vi "Text control 2 v7.1.vi"() -> ()   [LabVIEW 2016]
panel:
  in  "Tab Control":enum32{"Main", "Other parameters"}(tab)
  in  "Plot sample extrema vs time":bool
  out "Line running":i32
  out "Total lines":i32
  out "Path":path=path "C:/users/rlp38/09Apr2009LTtesting/test2.txt"
  out "I vs Vg":cluster{"Y data in":dbl[], "X data in":dbl[]}[](graph)
  out "Is max":dbl format="%.2e"
  out "Id max":dbl format="%.2e"
  out "Ig max":dbl format="%.2e"
  out "Imax vs time":cluster{"Y data in":dbl[], "X data in":dbl[]}[](graph)
  out "Imin vs time":cluster{"Y data in":dbl[], "X data in":dbl[]}[](graph)
  out "I vs Vd":cluster{"Y data in":dbl[], "X data in":dbl[]}[](graph)
  in  "Script":string="#pulsedstressV d 0.03 20 0 0.5 0.0827 5\n#\n#itime m\n#gaterangemode a\n#drainrangemode a\n#pulsed on 0.05 0 0.02\n#transfer d -10 40 1 5 40 35\n#transfer d -10 40 1 5 40 35\n#transfer d -10 40 1 5 40 35\n#output d 0 40 20 0 40 1\n#\n#\n#sample 1 0.008 221 6 0.003\n#samplei 400e-6 200 6 0.002 0.1\n#vsu2pulse -10 4\n#\n#stressV 0.016 0.03 2e-4 0.1e-3 11\n#stressI 220e-7 0.08 15\n#transfer s -1 1 0.5 -0.005 0.005 0.005\n#output s 0 0 0 -0.008 0.008 0.002"
  out "Command running:":string
  out "Serial port data":string
  out "Elapsed Time":dbl caption="Elapsed Time (s)"
  in  "Time Units":u16(ring)=1 items=["Seconds", "Minutes", "Hours"]
  in  "Time Offset":dbl caption="Set Start Time (s)"
  in  "Reset":bool
  in  "Auto Reset":bool
  in  "integration time":u32(slide) max=2 step=1 scale=0.0..2.0
  out "Is on":dbl format="%.2e"
  out "Id on":dbl format="%.2e"
  out "Ig on":dbl format="%.2e"
  out "Ion vs time":cluster{"Y data in":dbl[], "X data in":dbl[]}[](graph)
  out "Ioff vs time":cluster{"Y data in":dbl[], "X data in":dbl[]}[](graph)
  out "Ig min":dbl format="%.2e"
  out "Id min":dbl format="%.2e"
  out "Is min":dbl format="%.2e"
  out "Is off":dbl format="%.2e"
  out "Id off":dbl format="%.2e"
  out "Ig off":dbl format="%.2e"
  in  "Integration time (long)":dbl=0.32 min=0.04 max=2.0 step=0.02 format="%.2f"
  in  "Integration time (short)":dbl=0.0019 min=8e-05 max=0.0019 step=8e-05 format="%^.0e"
  in  "Drain: Compliance":dbl=0.001 format="%.8f"
  in  "Gate: Compliance":dbl=0.001 format="%.8f"
  in  "Interrupt scan":bool
  in  "Interrupt program":bool
  in  "Plot output curve extrema vs time":bool
  in  "Plot transfer curve extrema vs time":bool
  out "I vs time (Bias Stress)":cluster{"Y data in":dbl[], "X data in":dbl[]}[](graph)
  in  "Sample I - Probe 4 (Disabled)":u32(ring)=3 items=["SMU1  ", "SMU2  ", "SMU3  ", "SMU4  ", "SMU5  ", "SMU6  ", "VSU1  ", "VSU2  "]
  in  "Sample I - Source/Common":u32(ring) items=["SMU1  ", "SMU2  ", "SMU3  ", "SMU4  ", "SMU5  ", "SMU6  ", "VSU1  ", "VSU2  "]
  in  "Sample I - Probe 3 (Disabled)":u32(ring)=2 items=["SMU1  ", "SMU2  ", "SMU3  ", "SMU4  ", "SMU5  ", "SMU6  ", "VSU1  ", "VSU2  "]
  in  "Sample I - Drain/Gate":u32(ring)=1 items=["SMU1  ", "SMU2  ", "SMU3  ", "SMU4  ", "SMU5  ", "SMU6  ", "VSU1  ", "VSU2  "]
  in  "Sample - Probe 4":u32(ring)=3 items=["SMU1  ", "SMU2  ", "SMU3  ", "SMU4  ", "SMU5  ", "SMU6  ", "VSU1  ", "VSU2  "]
  in  "Sample - Source/Common":u32(ring) items=["SMU1  ", "SMU2  ", "SMU3  ", "SMU4  ", "SMU5  ", "SMU6  ", "VSU1  ", "VSU2  "]
  in  "Sample - Gate":u32(ring)=2 items=["SMU1  ", "SMU2  ", "SMU3  ", "SMU4  ", "SMU5  ", "SMU6  ", "VSU1  ", "VSU2  "]
  in  "Sample - Drain":u32(ring)=1 items=["SMU1  ", "SMU2  ", "SMU3  ", "SMU4  ", "SMU5  ", "SMU6  ", "VSU1  ", "VSU2  "]
  in  "Gate Range\nmode":u16(ring) items=["Auto", "Limited", "Fixed"]
  in  "Gate Range":u8(slide)=3 max=11 scale=0.0..11.0
  in  "Source/Drain\nRange mode":u16(ring) items=["Auto", "Limited", "Fixed"]
  in  "Source/Drain Range":u8(slide)=3 max=11 scale=0.0..11.0
  in  "Panel Controls":T1={"Emergency Stop"=refnum, "TransGraph Max"=1e-05, "Text/Graph (text=false)"=TRUE} {"TransGraph Max" format="%.2e"}
  in  "Panel Controls 2":T2={"Emergency Stop"=refnum, "TransGraph Max"=1e-05, "Text/Graph (text=false)"=TRUE, "TransGraph Min"=1e-11} {"TransGraph Min" format="%.2e"; "TransGraph Max" format="%.2e"}
  out "error out":errorcluster
  in  "Delay before read (ms)":u32=1000
  in  "byte count":u32=64
  in  "Serial End Mode for Reads":u16(ring)=2 items=["None", "LastBit", "TermChar"]
  in  "Timeout (ms)":u32=10000
  in  "Enable Termination\nChar (T)":bool=TRUE
  in  "Termination char\n(0xA = '\\n' = LF)\n(0xD = '\\r' = CR)":u8=13 format="%.0x"
  in  "flow control":u16(ring) items=["None"=0, "XON/XOFF"=1, "RTS/CTS"=2, "DTR/DSR"=4]
  in  "stop bits":u16(ring)=10 items=["1.0"=10, "1.5"=15, "2.0"=20]
  in  "parity":u16(ring) items=["None", "Odd", "Even", "Mark", "Space"]
  in  "data bits":u16=8 min=5 max=8 step=1
  in  "VISA resource name":refnum<visa-resource-name>="COM6"
  in  "baud rate":u32=9600
  out "Timings Indicator":T3
  in  "Timings (overwritten by the Front Panel)":T4={"integration time"=0, "Short/Long integration time"=0.00064, "hold time (sec)"=0.0, "delay time (sec)"=0.0, "Step Time (0 disables)"=0.0, "sweep method"=0, "Pulse period"=0.005, "Base voltage"=0.0, "Pulse width"=0.0005} {"Pulse width" min=0.0005 max=0.1 step=0.0001 format="%.4f"; "Base voltage" format="%^.4e"; "Pulse period" min=0.005 max=1.0 step=0.0001 format="%.4f"; "sweep method" items=["Continuous", "Pulsed"]; "Step Time (0 disables)" format="%.2f"; "delay time (sec)" format="%.4f"; "hold time (sec)" format="%.4f"; "Short/Long integration time" format="%^.0e"; "integration time" scale=0.0..2.0}
  in  "Probe 4":cluster{"on/off":bool, "Voltage":dbl} {"Voltage" min=-100.0 max=100.0 format="%.2f"}
  in  "Full Reset":bool
  in  "Standby":T5
  out "Probe 4 Indicator":cluster{"on/off":bool, "Voltage":dbl} {"Voltage" min=-100.0 max=100.0 format="%.2f"}
  in  "Transfer/Output - Drain":u32(ring)=1 items=["SMU1  ", "SMU2  ", "SMU3  ", "SMU4  ", "SMU5  ", "SMU6  ", "VSU1  ", "VSU2  "]
  in  "Transfer/Output - Gate":u32(ring)=2 items=["SMU1  ", "SMU2  ", "SMU3  ", "SMU4  ", "SMU5  ", "SMU6  ", "VSU1  ", "VSU2  "]
  in  "Transfer/Output - Source/Common":u32(ring) items=["SMU1  ", "SMU2  ", "SMU3  ", "SMU4  ", "SMU5  ", "SMU6  ", "VSU1  ", "VSU2  "]
  in  "Transfer/Output - Probe 4":u32(ring)=3 items=["SMU1  ", "SMU2  ", "SMU3  ", "SMU4  ", "SMU5  ", "SMU6  ", "VSU1  ", "VSU2  "]
  in  "Pulsed Stress V - Probe 4":u32(ring)=3 items=["SMU1  ", "SMU2  ", "SMU3  ", "SMU4  ", "SMU5  ", "SMU6  ", "VSU1  ", "VSU2  "]
  in  "Pulsed Stress V - Vextra":u32(ring)=7 items=["SMU1  ", "SMU2  ", "SMU3  ", "SMU4  ", "SMU5  ", "SMU6  ", "VSU1  ", "VSU2  "]
  in  "Pulsed Stress V - Drain":u32(ring)=1 items=["SMU1  ", "SMU2  ", "SMU3  ", "SMU4  ", "SMU5  ", "SMU6  ", "VSU1  ", "VSU2  "]
  in  "Pulsed Stress V - Source/Common":u32(ring) items=["SMU1  ", "SMU2  ", "SMU3  ", "SMU4  ", "SMU5  ", "SMU6  ", "VSU1  ", "VSU2  "]
  in  "Pulsed Stress V - Gate":u32(ring)=2 items=["SMU1  ", "SMU2  ", "SMU3  ", "SMU4  ", "SMU5  ", "SMU6  ", "VSU1  ", "VSU2  "]
  in  "FPP - Drain":u32(ring)=1 items=["SMU1  ", "SMU2  ", "SMU3  ", "SMU4  ", "SMU5  ", "SMU6  ", "VSU1  ", "VSU2  "]
  in  "FPP - Gate":u32(ring)=2 items=["SMU1  ", "SMU2  ", "SMU3  ", "SMU4  ", "SMU5  ", "SMU6  ", "VSU1  ", "VSU2  "]
  in  "FPP - Probe 1":u32(ring) items=["SMU1  ", "SMU2  ", "SMU3  ", "SMU4  ", "SMU5  ", "SMU6  ", "VSU1  ", "VSU2  "]
  in  "FPP - Probe 2":u32(ring)=3 items=["SMU1  ", "SMU2  ", "SMU3  ", "SMU4  ", "SMU5  ", "SMU6  ", "VSU1  ", "VSU2  "]
  in  "FPP - Source":u32(ring)=6 items=["SMU1  ", "SMU2  ", "SMU3  ", "SMU4  ", "SMU5  ", "SMU6  ", "VSU1  ", "VSU2  "]
  in  "Stress V - Drain":u32(ring)=1 items=["SMU1  ", "SMU2  ", "SMU3  ", "SMU4  ", "SMU5  ", "SMU6  ", "VSU1  ", "VSU2  "]
  in  "Stress V - Gate":u32(ring)=2 items=["SMU1  ", "SMU2  ", "SMU3  ", "SMU4  ", "SMU5  ", "SMU6  ", "VSU1  ", "VSU2  "]
  in  "Stress V - Source/Common":u32(ring) items=["SMU1  ", "SMU2  ", "SMU3  ", "SMU4  ", "SMU5  ", "SMU6  ", "VSU1  ", "VSU2  "]
  in  "Stress I - Drain/Gate":u32(ring)=1 items=["SMU1  ", "SMU2  ", "SMU3  ", "SMU4  ", "SMU5  ", "SMU6  ", "VSU1  ", "VSU2  "]
  in  "Stress I - Source/Common":u32(ring) items=["SMU1  ", "SMU2  ", "SMU3  ", "SMU4  ", "SMU5  ", "SMU6  ", "VSU1  ", "VSU2  "]
  in  "VSU2 Stress - Source/Common":u32(ring) items=["SMU1  ", "SMU2  ", "SMU3  ", "SMU4  ", "SMU5  ", "SMU6  ", "VSU1  "]
  in  "VISA resource name in":refnum<visa-resource-name>="GPIB0::14::INSTR"
  in  "Gate":T6={"Gate Start"=0.0, "Gate Stop"=2.0, "Gate Step (linear only)"=1.0, "Gate Compliance"=0.0001, "Gate PComp"=0.0, "Range mode"=0, "Range"=6} {"Range" max=11 scale=0.0..11.0; "Range mode" items=["Auto", "Limited", "Fixed"]; "Gate PComp" format="%^.2e"; "Gate Compliance" format="%^.2e"; "Gate Step (linear only)" format="%^.4e"; "Gate Stop" format="%^.4e"; "Gate Start" format="%^.4e"}
  in  "Drain 2":T7={"Drain Start"=0.0, "Drain Stop"=2.0, "Drain Compliance"=0.0001, "Drain Step"=1.0, "Drain PComp"=0.0, "Range mode"=0, "Range"=6} {"Range" max=11 scale=0.0..11.0; "Range mode" items=["Auto", "Limited", "Fixed"]; "Drain PComp" format="%^.2e"; "Drain Step" format="%^.4e"; "Drain Compliance" format="%^.2e"; "Drain Stop" format="%^.4e"; "Drain Start" format="%^.4e"}
  # "Time"
  # "Syntax:\nitime [s|m|l] time(sec): [s|m|l] determines the integration time setting (small|medium|long) and time sets the value.\nNOTE: The value of the integration time has to be within the range allowed by its category (s|m|l), otherwise, the closest value will be used. (e.g. if the category is set to short but the time value is very long, the actual value used will be the maximum short integration time.\nIntegration times:\n    Short: Default: 640 us. Range: 8E-5 - 1.92E-3 seconds.\n    Medium: Fixed at 1 NPL cycle (0.02 seconds).\n    Long: Default: 16 NPL cycles (0.32 seconds). Range: 2-100 NPL cycles (0.04 seconds - 2 seconds).\ngaterangemode [a|l|f]\ndrainrangemode [a|l|f]\npulsed [on|off] PulsePeriod(sec) PulseBaseVoltage PulseONWidth(sec)\nstandby [on l off]\nwait NumMilliseconds\nwait-min NumMinutes\n# texthere = comment\nProbe4 [ON|OFF] Voltage\ntransfer [s|d] VgStart VgStop VgStep VdStart VdStop VdStep\noutput [s|d] VgStart VgStop VgStep VdStart VdStop VdStep\nsample Vg Vd NumSamples Time(s) SampleInterval(s)\nsamplei Idg NumSamples Time(s) SampleInterval(s) VDGcompliance\n100 samples is approximately 13 seconds with medium integration\n# if in doubt use SampleInterval(s) = 0.004\n    NOTE: When doing bias stress measurements, it is best to set the Time Units to \"Seconds\", as the \"sample\" command has been configured to give the output to seconds.\nstressV VG VD IGcompliance IDcompliance Duration(sec)\nstressI IDG VDGcompliance Duration(sec)\nvsu2pulse Bias Duration(s)\npulsedstressV [s|d] VEstop VgON VgOFF Period(s) PulseONwidth(s) Vd\nsample-fpp Vg Vd NumSamples Time\nresample-fpp Vg Vd\ntransfer-fpp [s|d] VgStart VgStop VgStep VdStart VdStop VdStep\noutput-fpp [s|d] VgStart VgStop VgStep VdStart VdStop VdStep\nserial SerialPortCommand"
  # "1\n2\n3\n4\n5\n6\n7\n8\n9\n10\n11\n12\n13\n14\n15\n16\n17\n18\n19\n20"
  # "SMUs"
  # "Serial port settings"
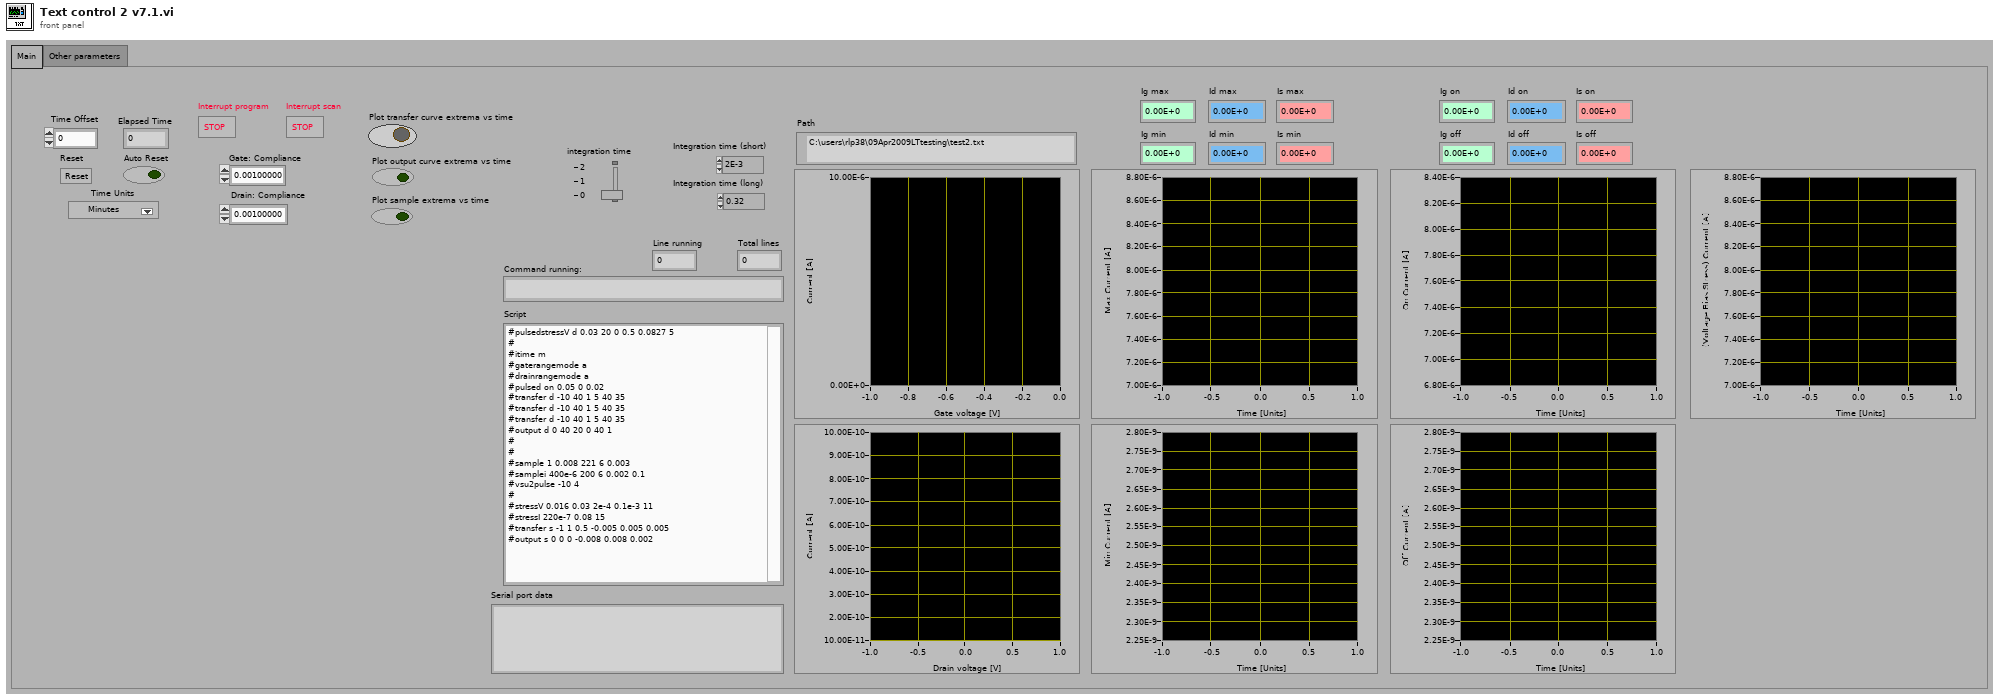
[diagram p1: front panel]
types:
  T1 = cluster{"Emergency Stop":refnum<vi>, "TransGraph Max":dbl, "Text/Graph (text=false)":bool}
  T2 = cluster{"Emergency Stop":refnum<vi>, "TransGraph Max":dbl, "Text/Graph (text=false)":bool, "TransGraph Min":dbl}
  T3 = cluster{"integration time (0:s, 1:m, 2:l)":u32, "Short/Long integration time":dbl, "hold time (sec)":dbl, "delay time (sec)":dbl, "Step Time (0 disables)":dbl, "sweep method":u16, "Pulse period":dbl, "Base voltage":dbl, "Pulse width":dbl}
  T4 = cluster{"integration time":u32, "Short/Long integration time":dbl, "hold time (sec)":dbl, "delay time (sec)":dbl, "Step Time (0 disables)":dbl, "sweep method":u16, "Pulse period":dbl, "Base voltage":dbl, "Pulse width":dbl}
  T5 = cluster{"Gate Standby":bool, "Drain Standby":bool}
  T6 = cluster{"Gate Start":dbl, "Gate Stop":dbl, "Gate Step (linear only)":dbl, "Gate Compliance":dbl, "Gate PComp":dbl, "Range mode":u16, "Range":u8}
  T7 = cluster{"Drain Start":dbl, "Drain Stop":dbl, "Drain Compliance":dbl, "Drain Step":dbl, "Drain PComp":dbl, "Range mode":u16, "Range":u8}
  T8 = enum16{"open", "replace", "create", "open or create", "replace or create", "replace or create with confirmation"}
  T9 = cluster{"V2 Start":dbl, "V2 Step":dbl, "Number of points":i32}
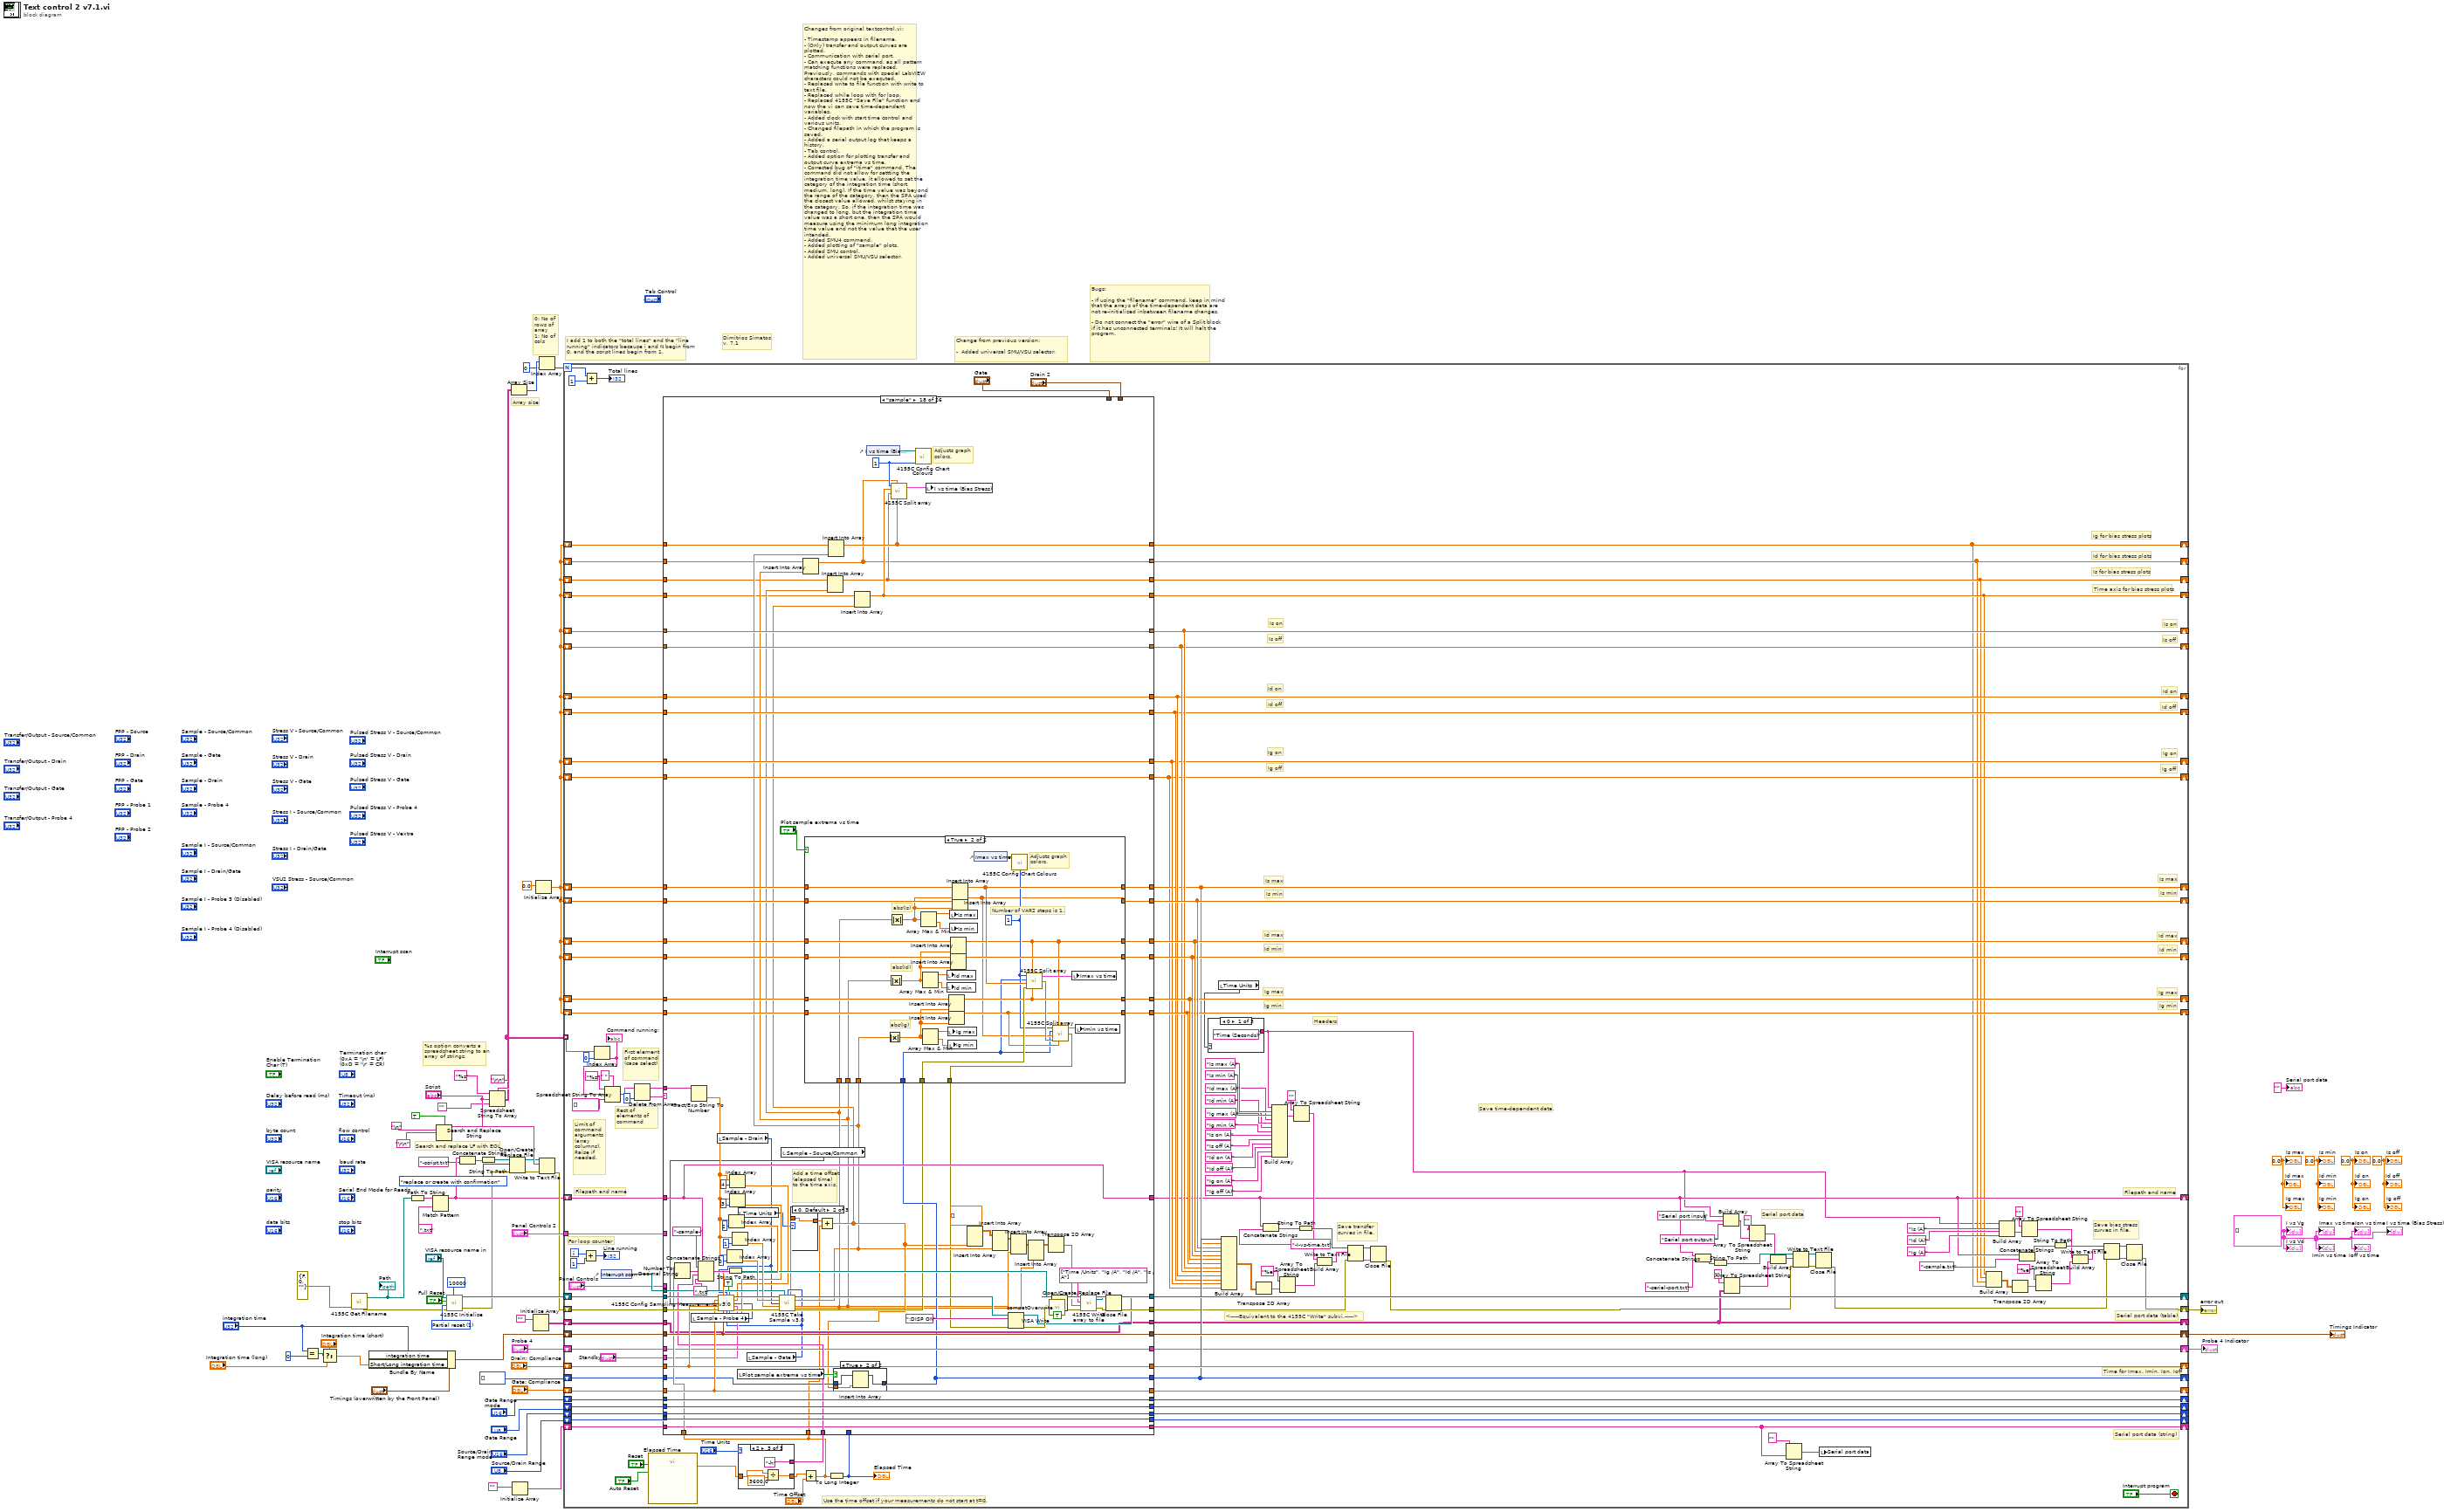
[diagram p0: block diagram]
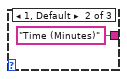
[diagram p2: hidden frame]
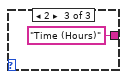
[diagram p3: hidden frame]
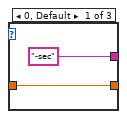
[diagram p4: hidden frame]
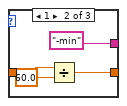
[diagram p5: hidden frame]
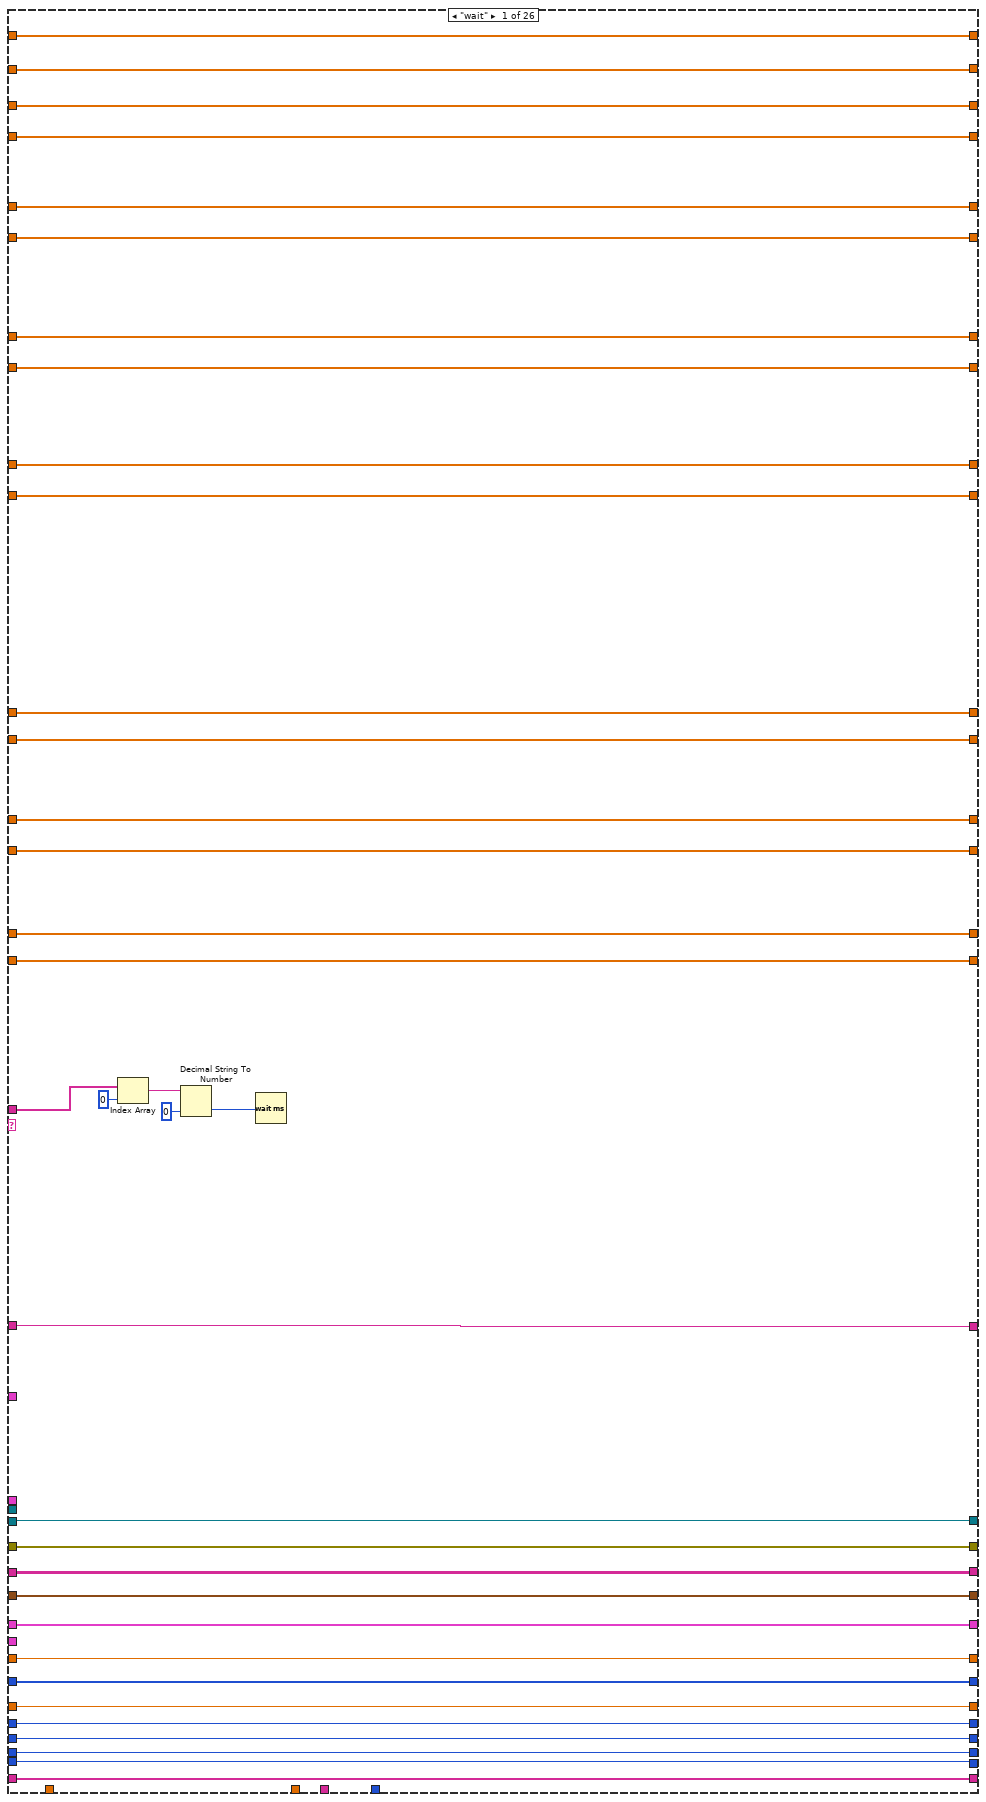
[diagram p6: hidden frame]
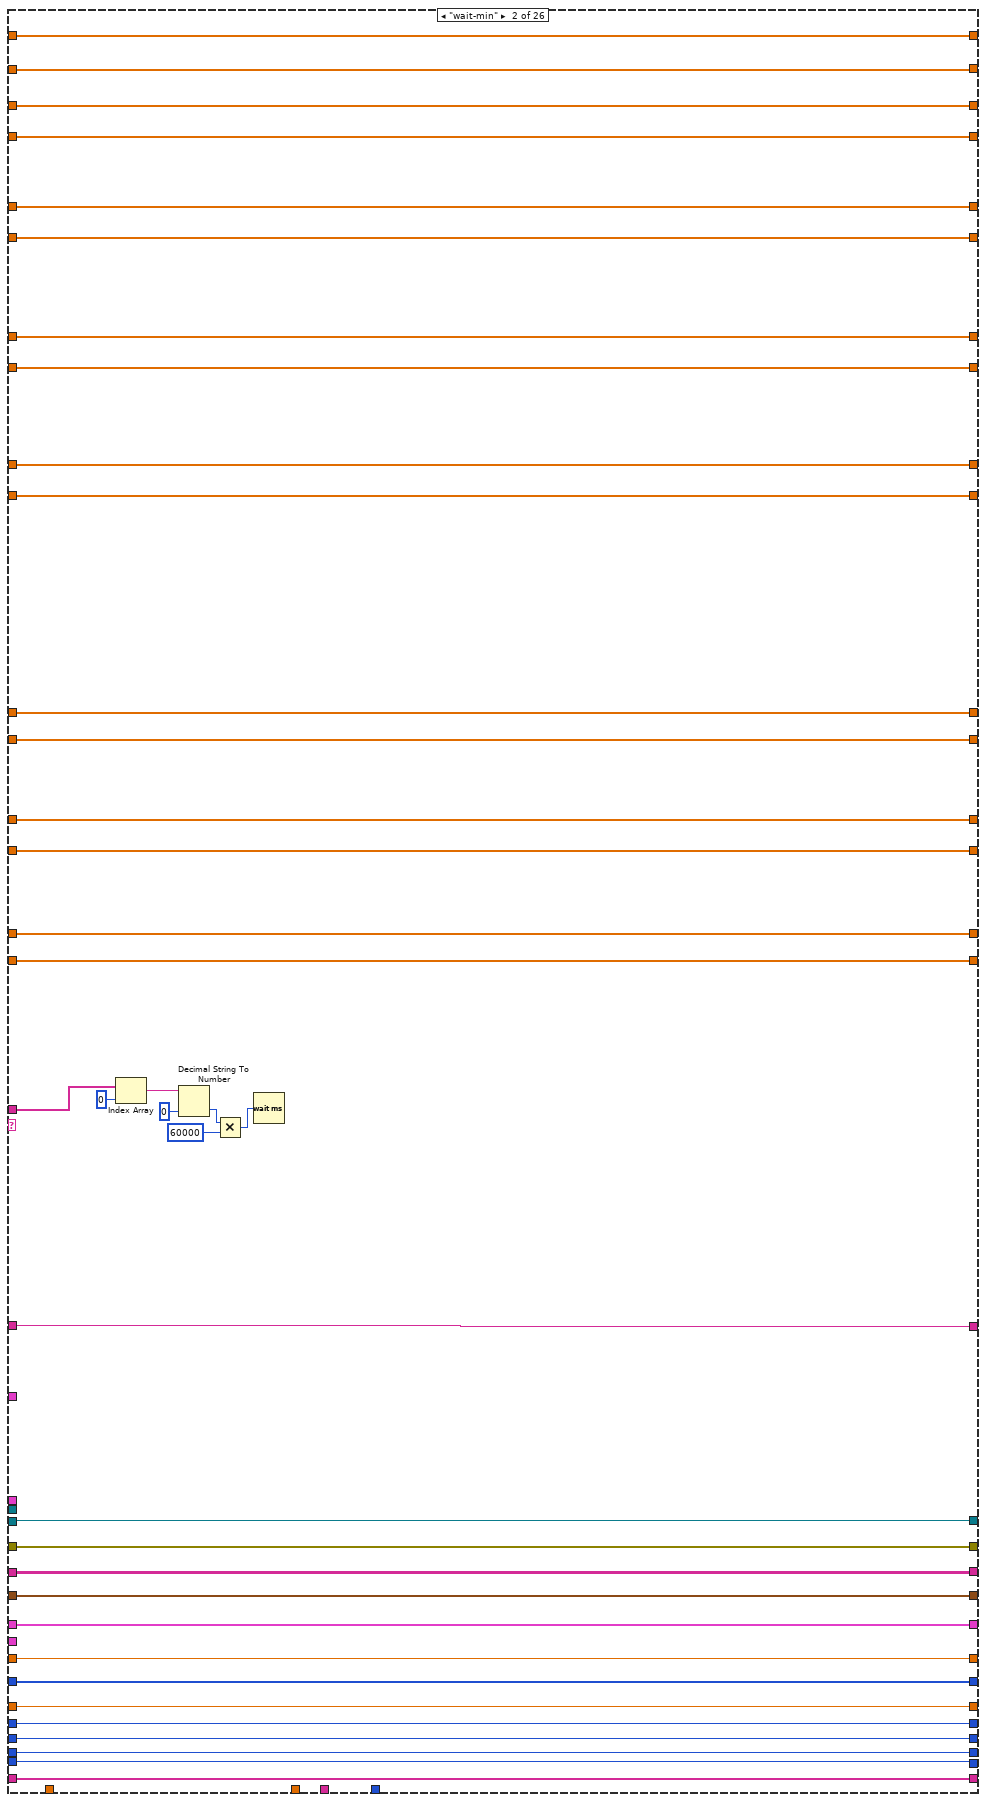
[diagram p7: hidden frame]
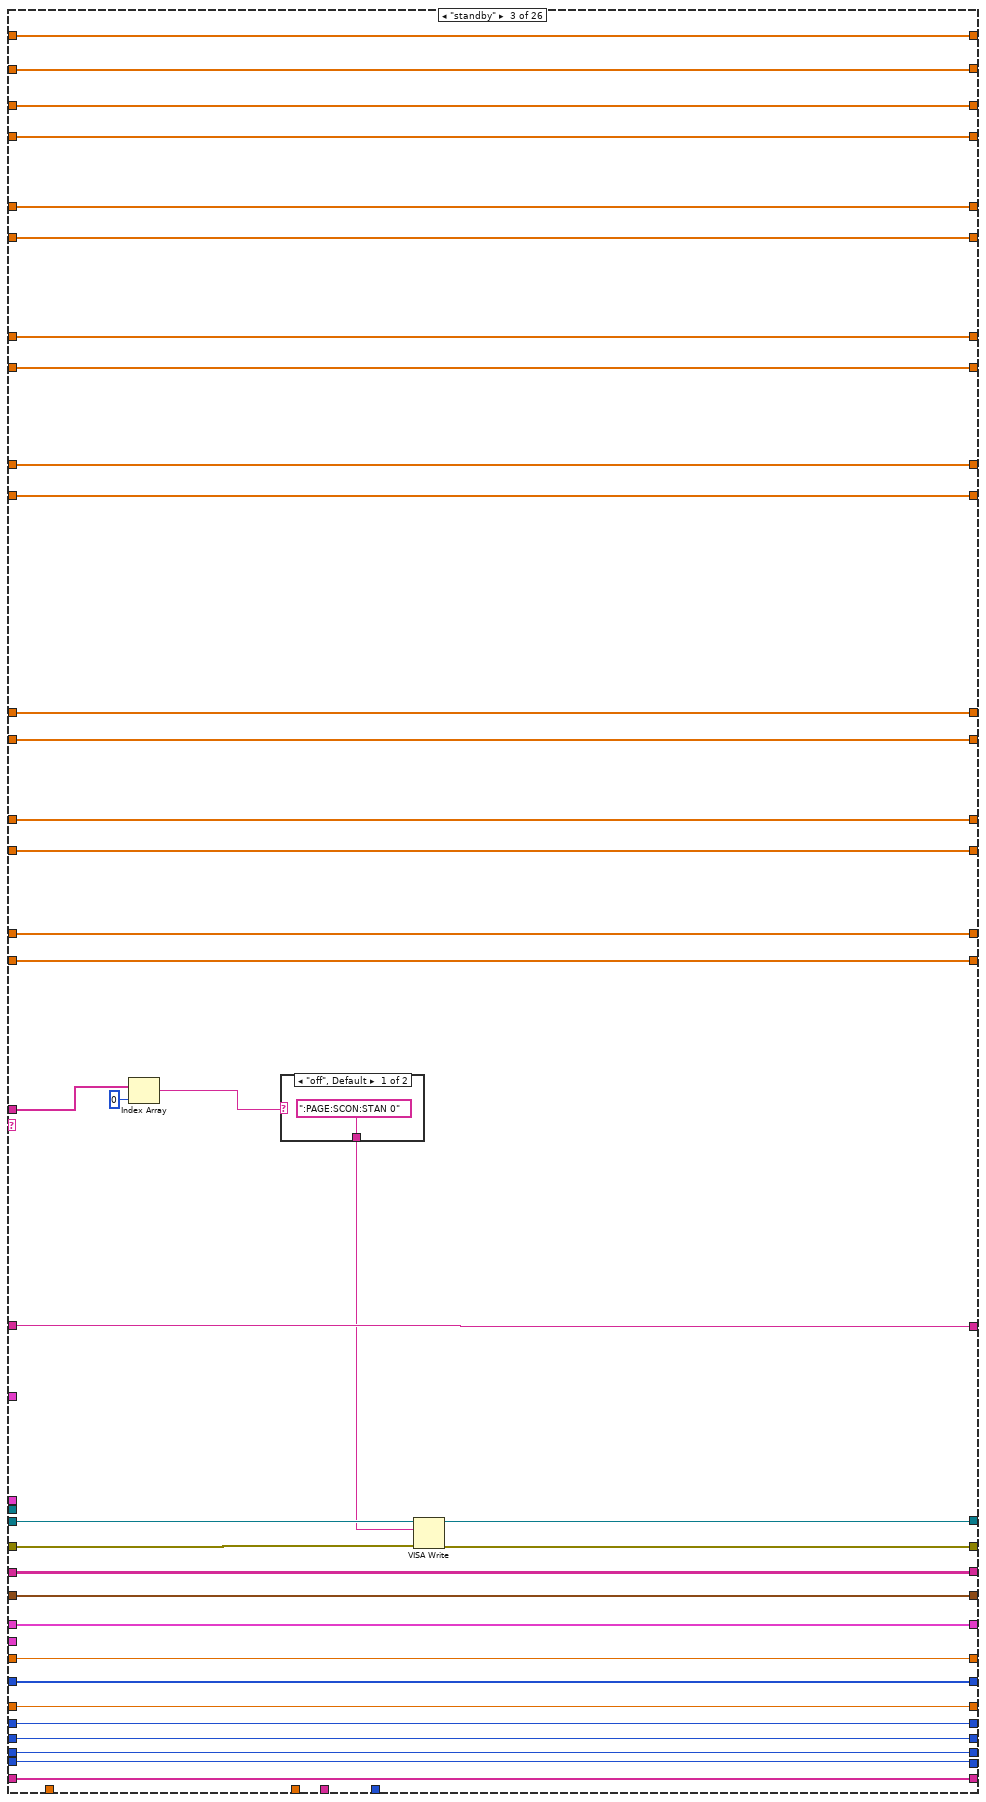
[diagram p8: hidden frame]
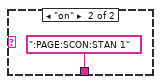
[diagram p9: hidden frame]
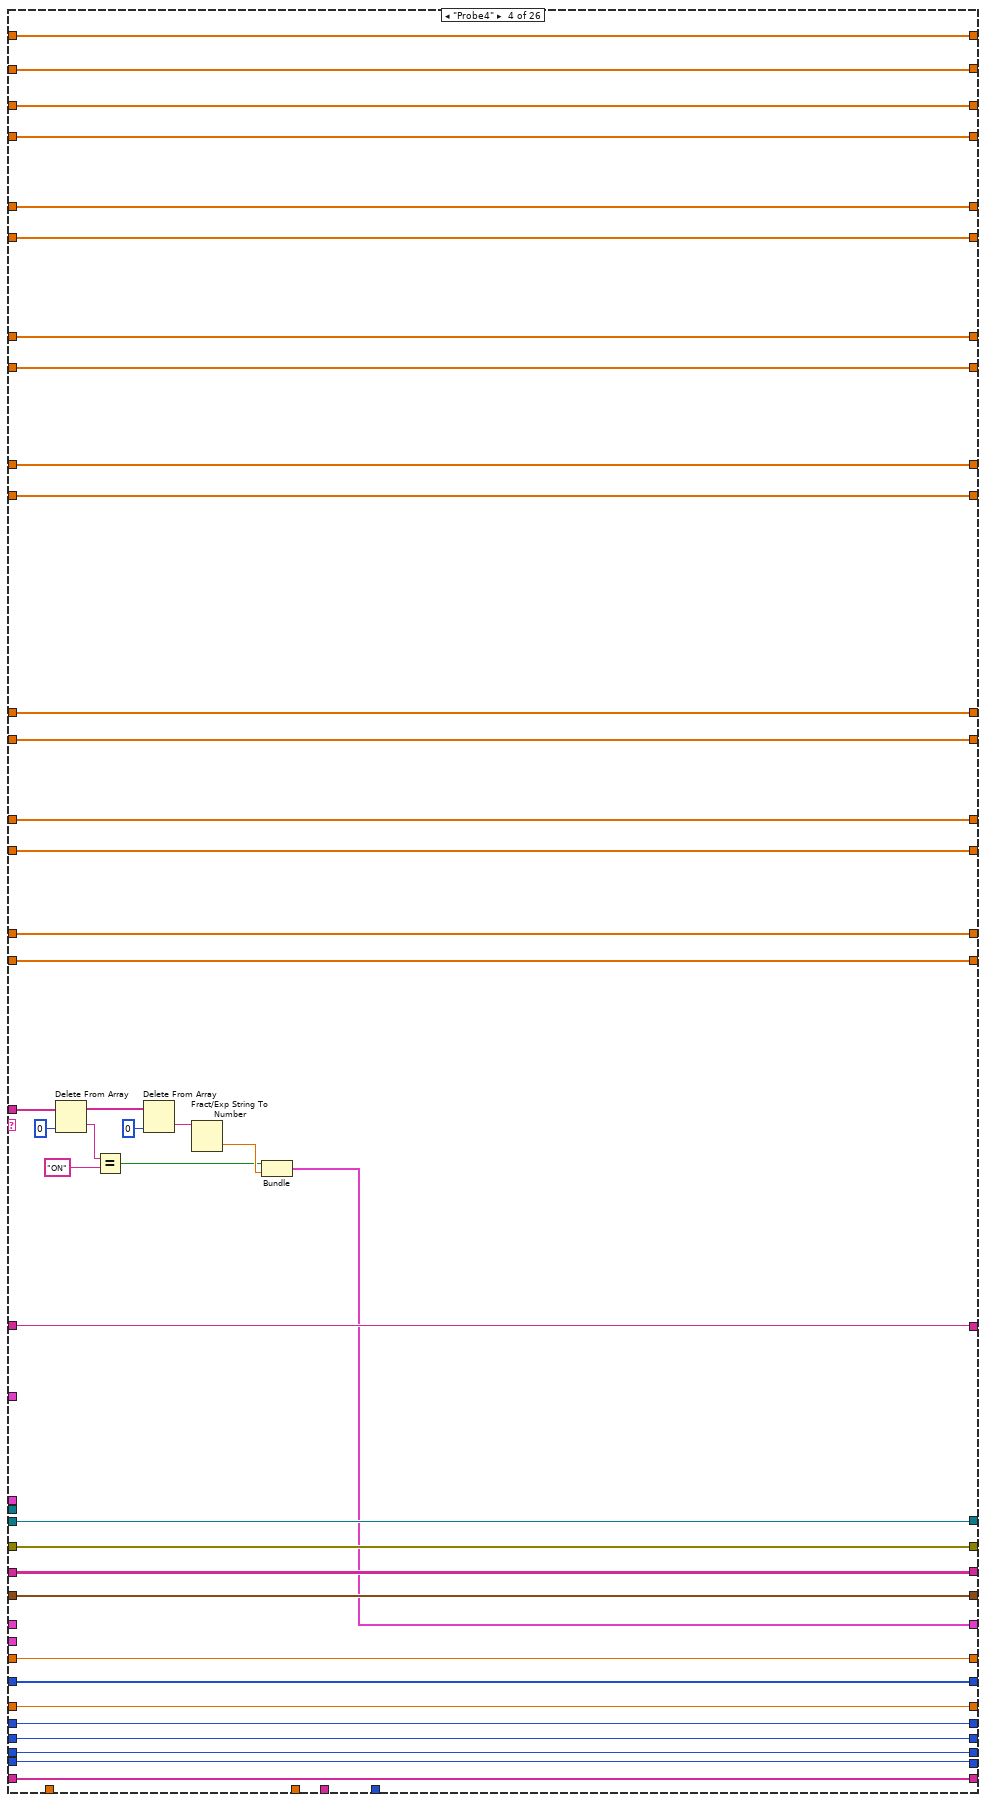
[diagram p10: hidden frame]
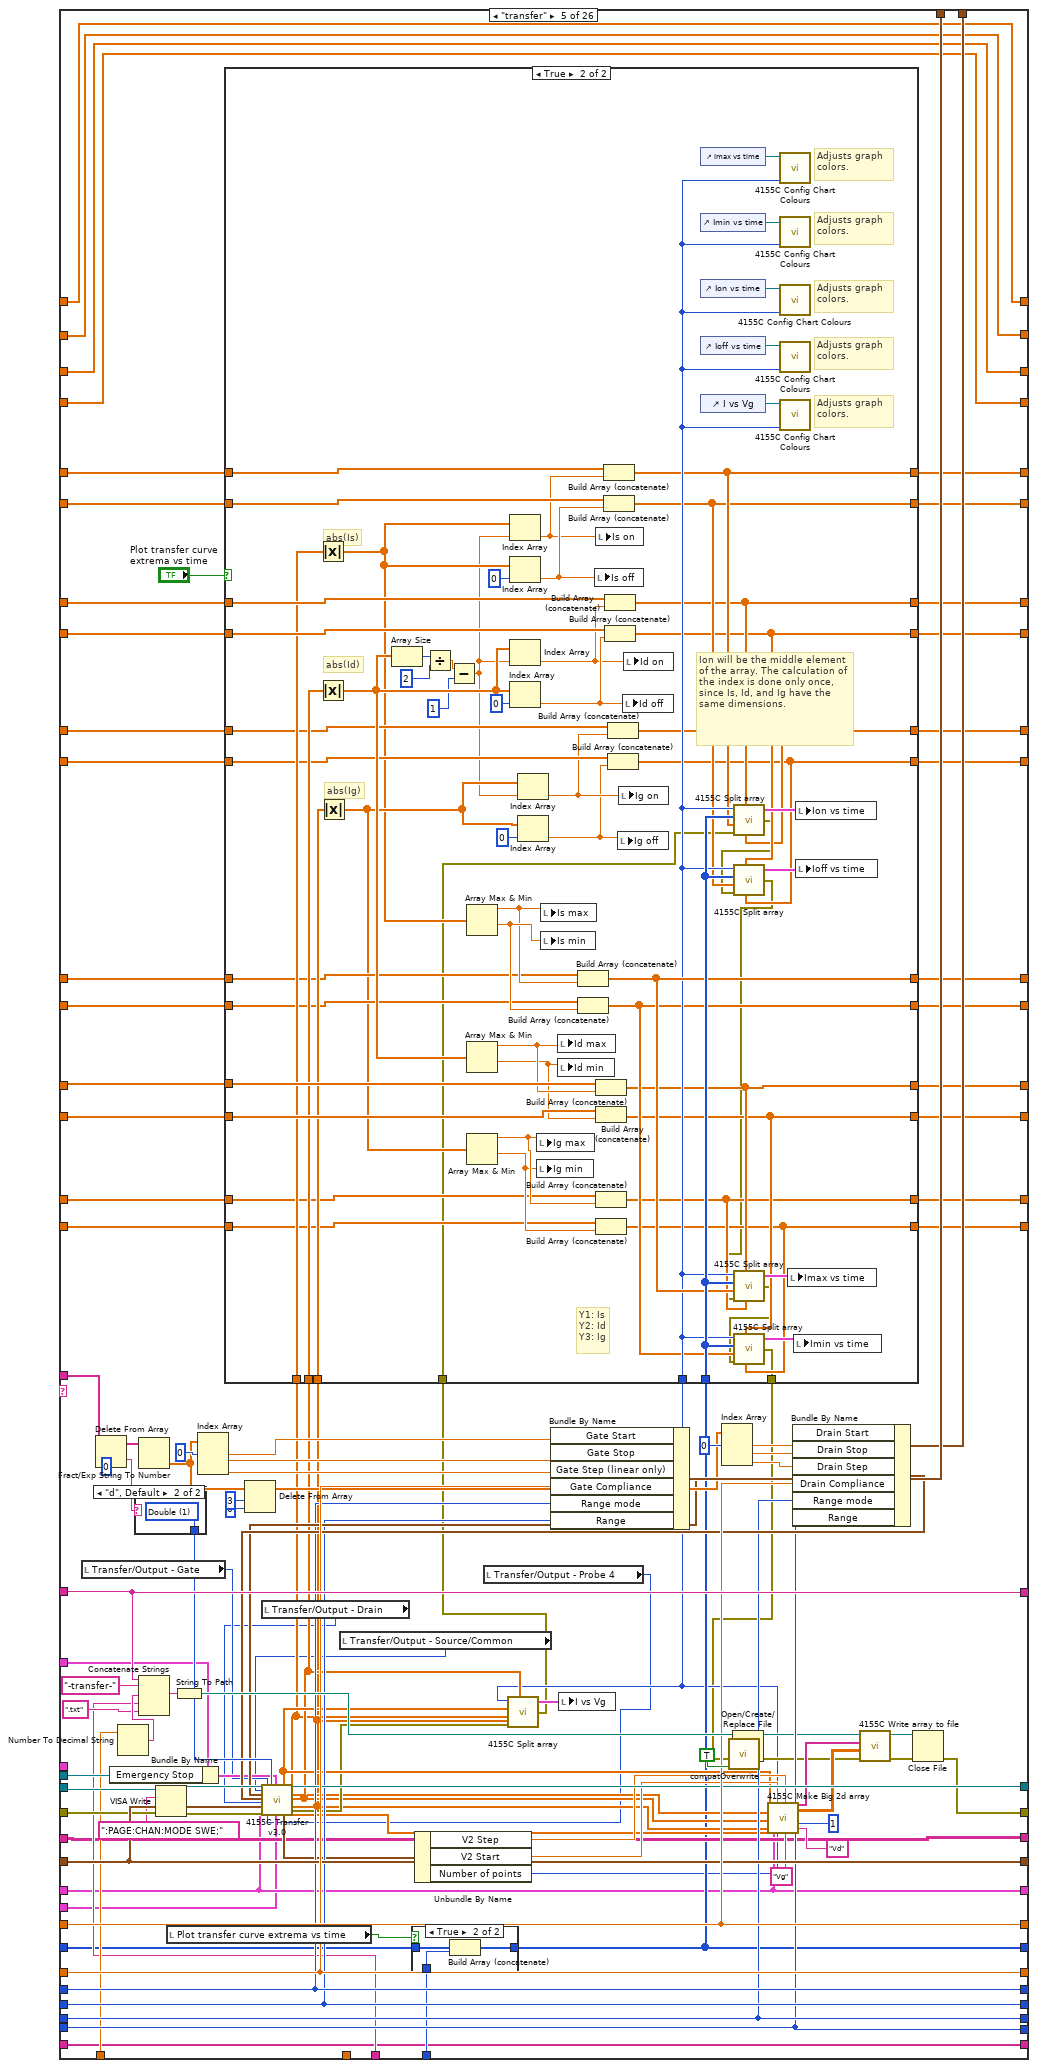
[diagram p11: hidden frame]
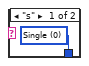
[diagram p14: hidden frame]
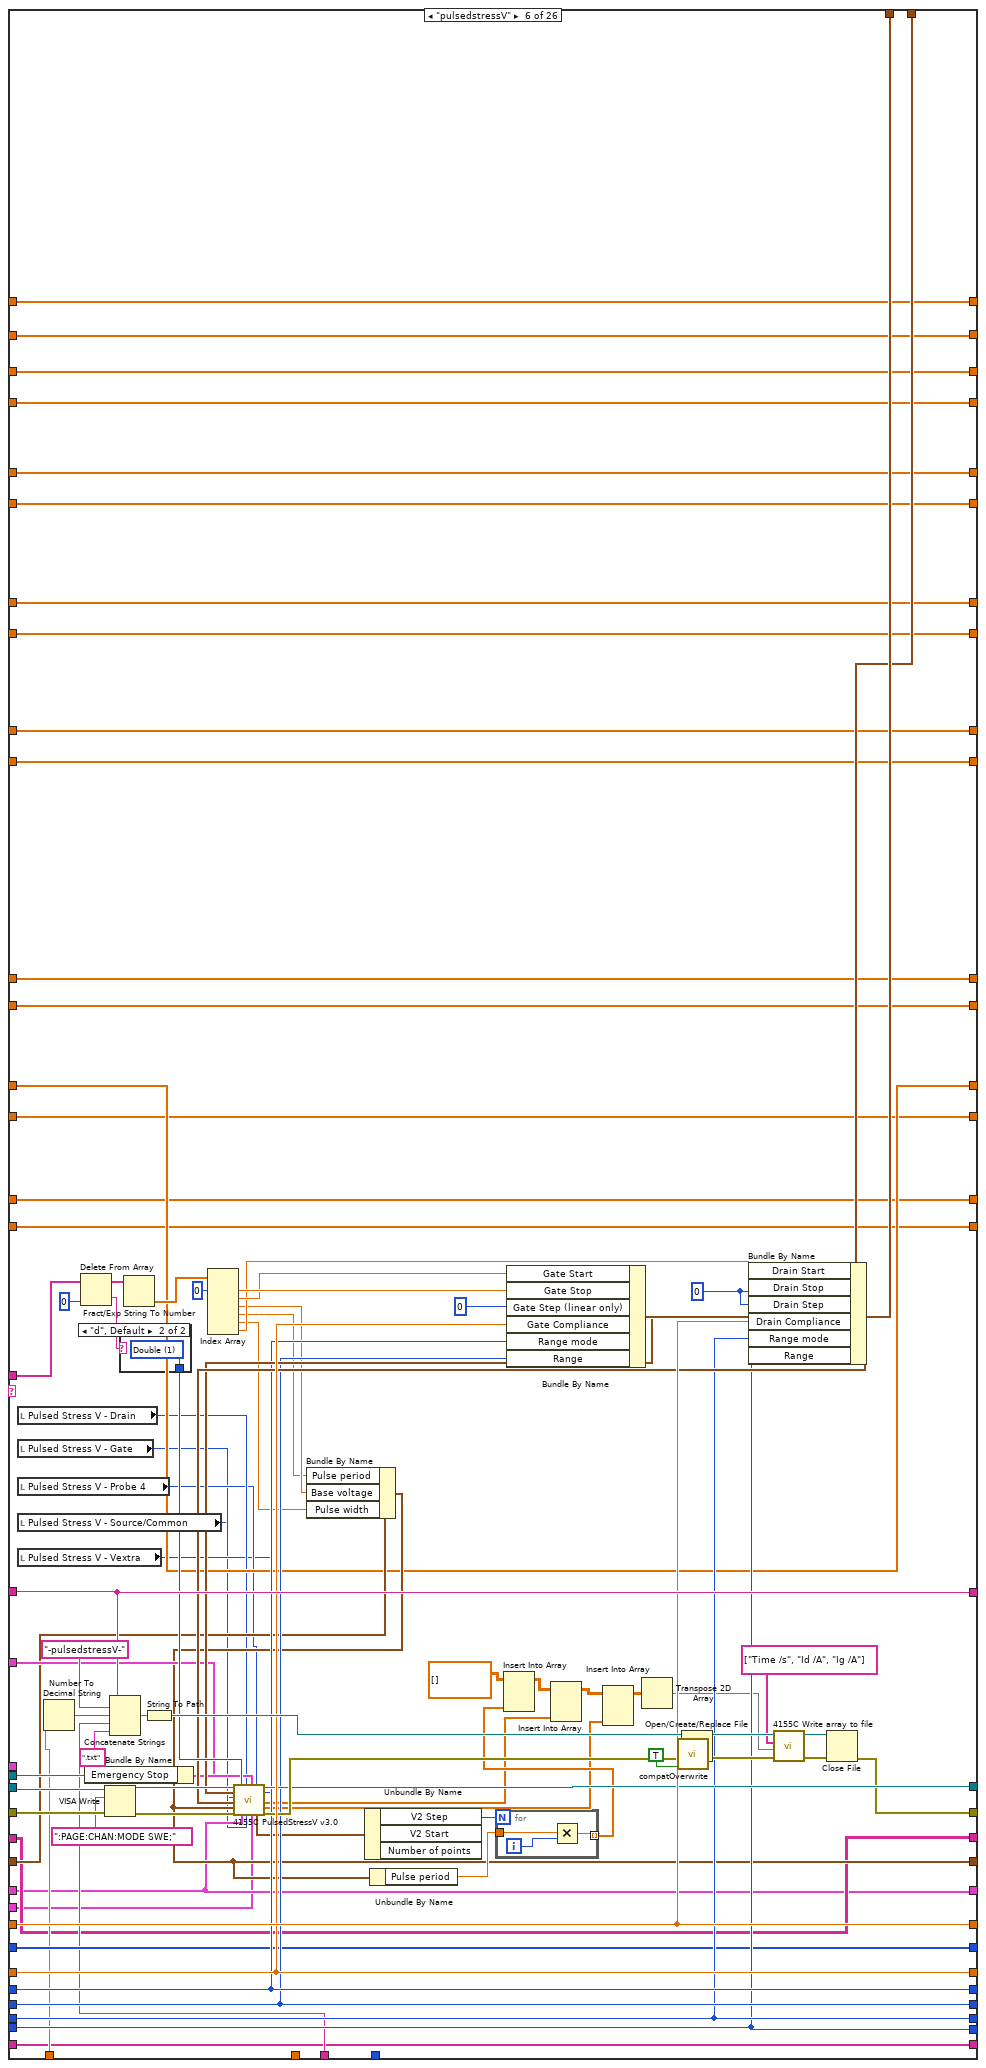
[diagram p15: hidden frame]
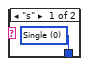
[diagram p16: hidden frame]
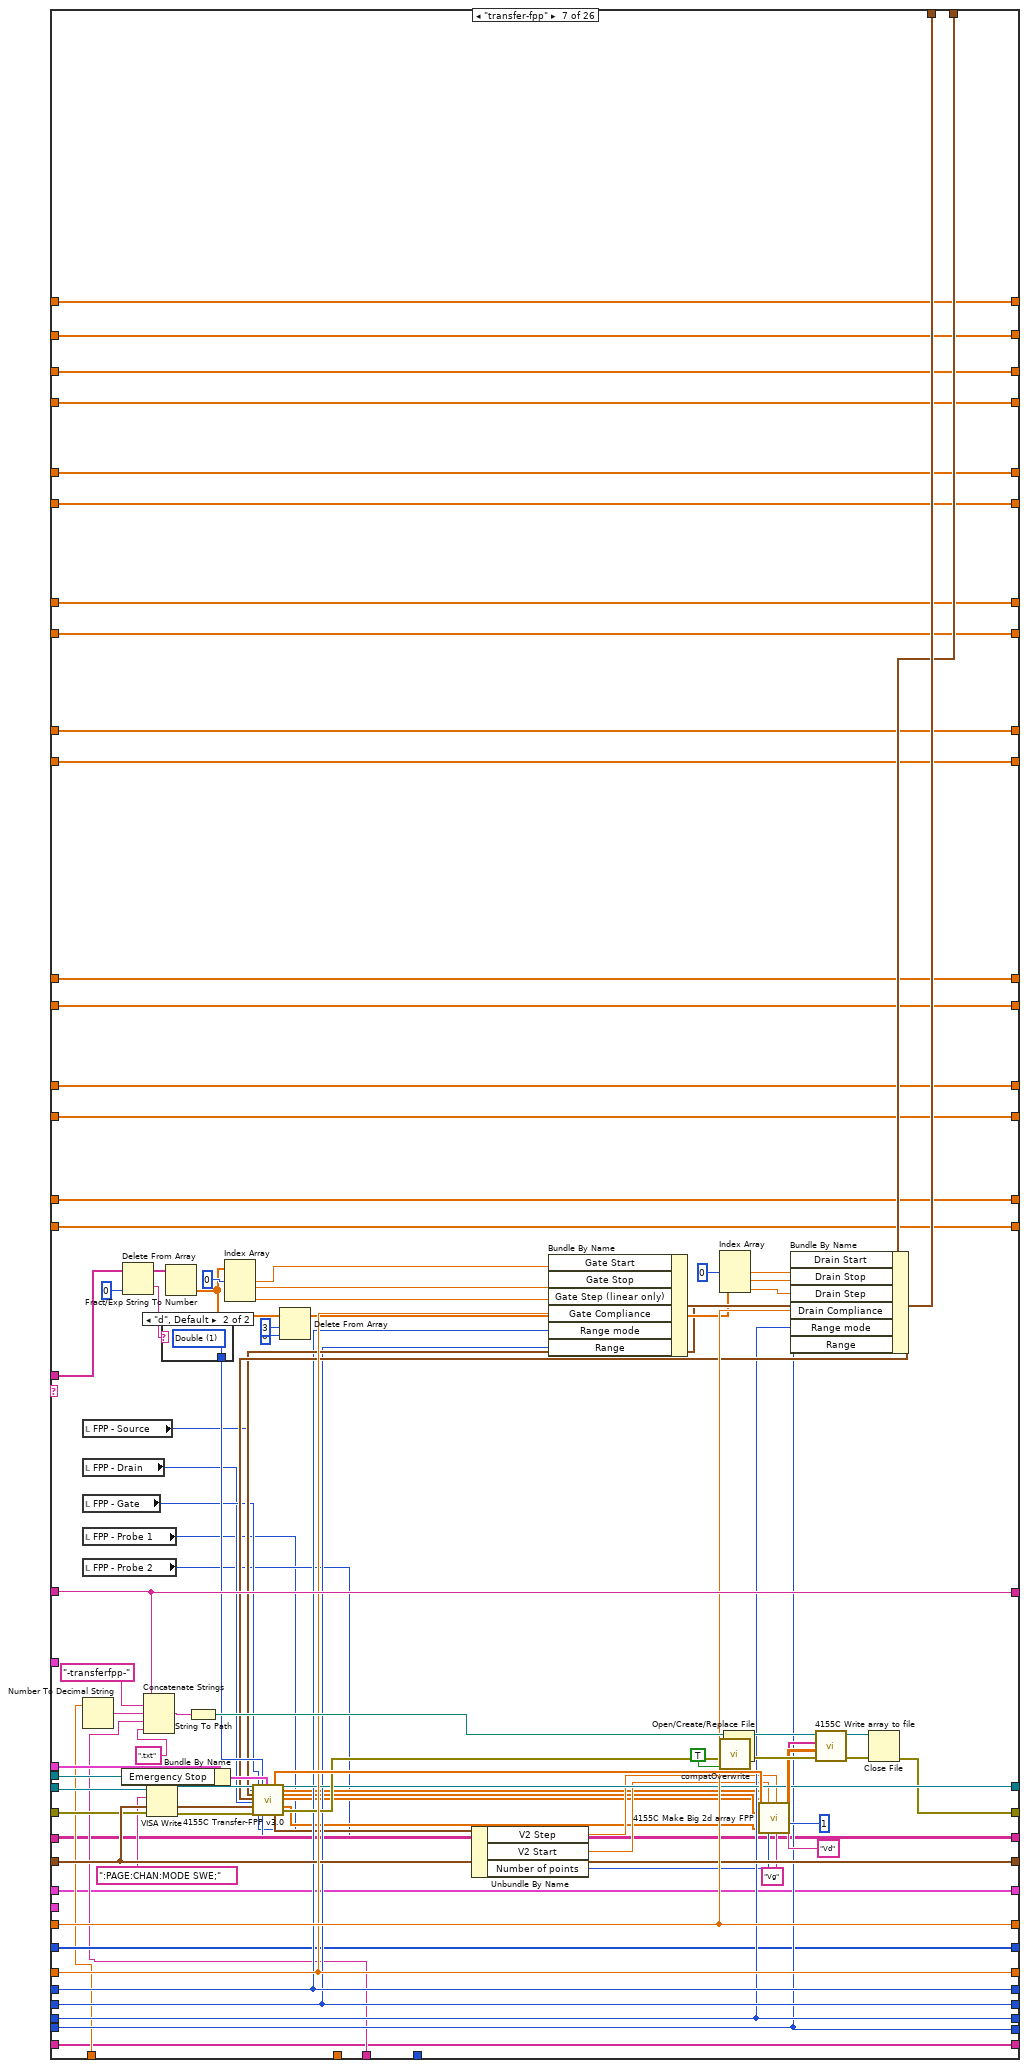
[diagram p17: hidden frame]
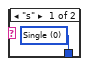
[diagram p18: hidden frame]
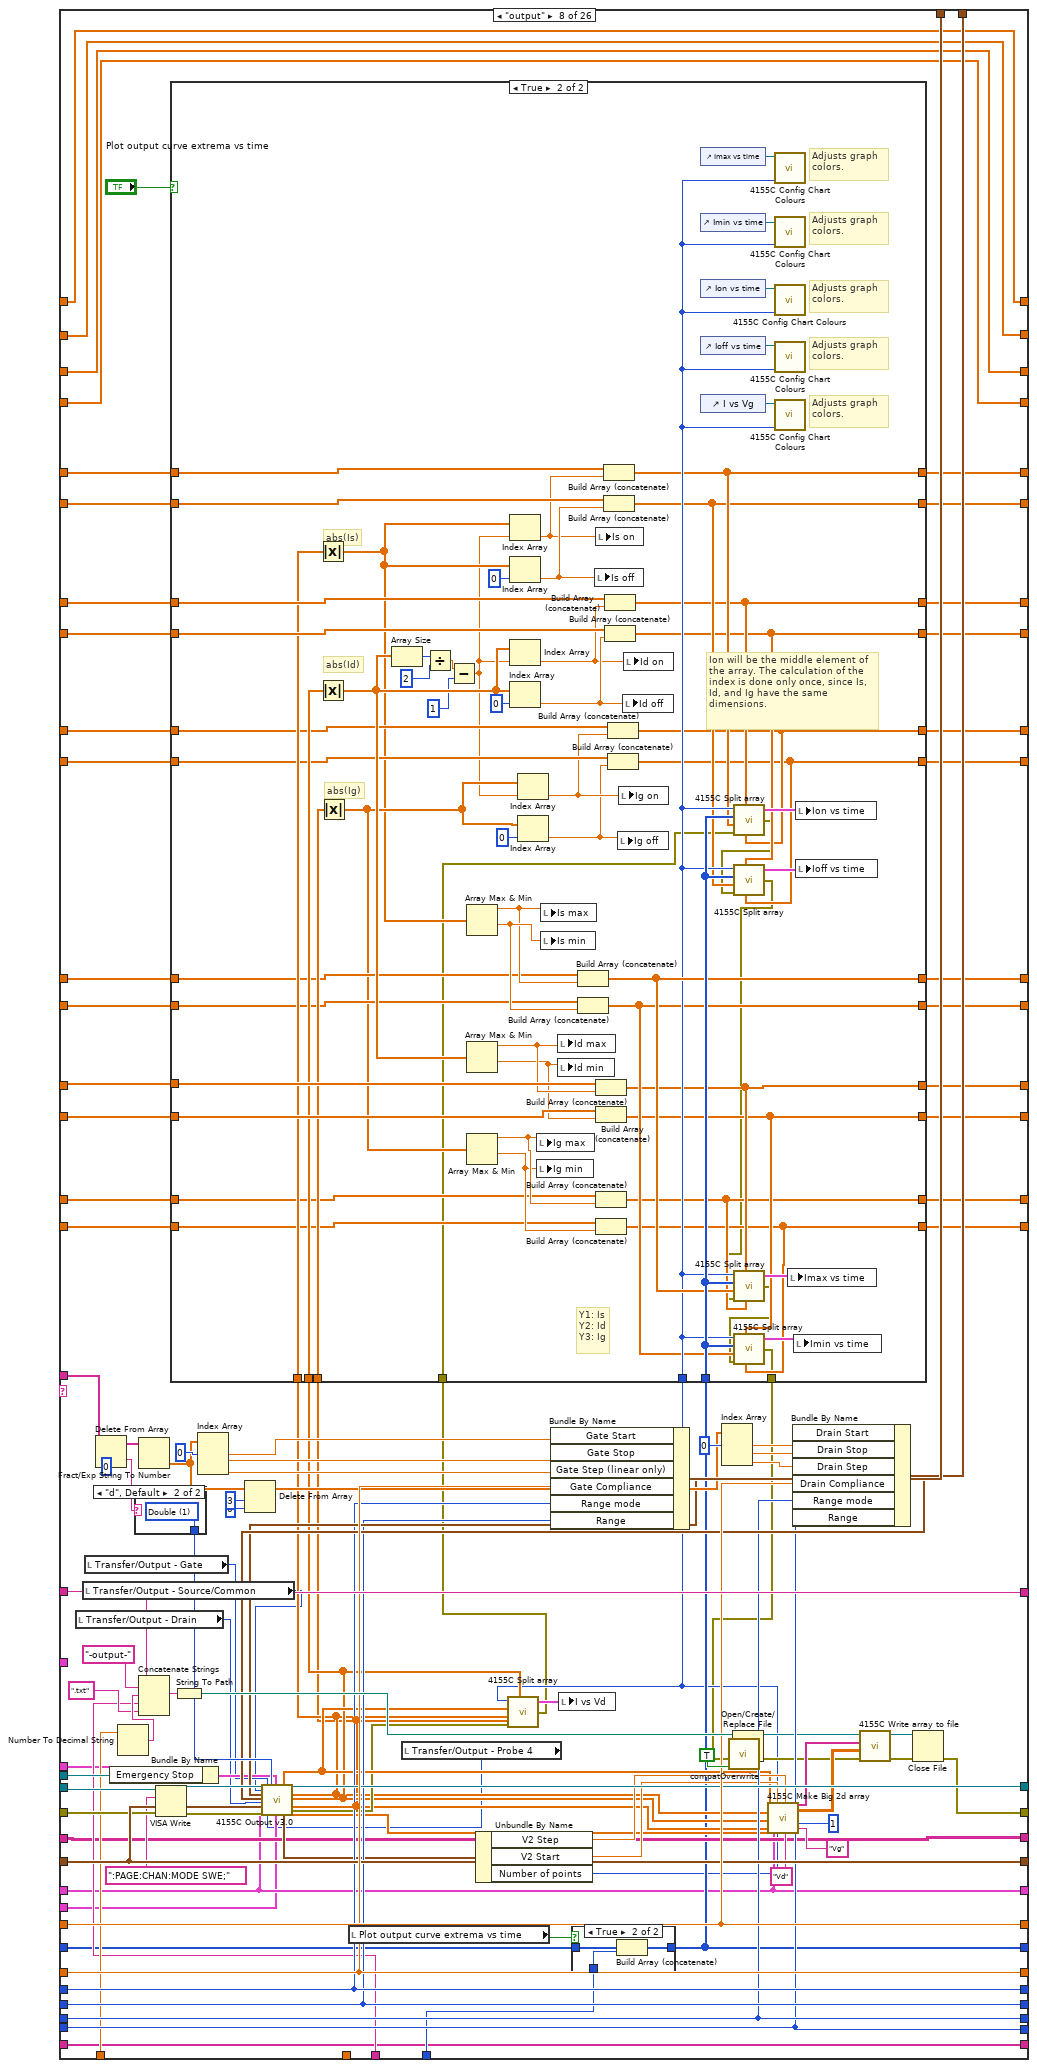
[diagram p19: hidden frame]
diagram:
  w2 = cluster{"Y data in":dbl[], "X data in":dbl[]}[] [] ("I vs Vg")
  w10 = 0.0 ("Is off")
  w11 = 0.0 ("Is on")
  w12 = 0.0 ("Is min")
  w13 = 0.0 ("Is max")
  w58 = u16 1 items=["Reset All", "Partial reset"] ("Type of reset")
  # "Change from previous version:\n\n-  Added universal SMU/VSU selector."
  # "I add 1 to both the \"total lines\" and the \"line running\" indicators because i and N begin from 0, and the script lines begin from 1."
  # "Bugs:\n\n- If using the \"filename\" command, keep in mind that the arrays of the time-dependent data are not re-initialized inbetween filename changes. \n\n- Do not connect the \"error\" wire of a Split block if it has unconnected terminals! It will halt the program."
  # "Array size"
  # "%s option converts a spreadsheet string to an array of strings."
  # "0: No of rows of array\n1: No of cols"
  # "Dimitrios Simatos\nv. 7.1"
  # "Changes from original textcontrol.vi:\n\n- Timestamp appears in filename.\n- (Only) transfer and output curves are plotted.\n- Communication with serial port.\n- Can execute any command, as all pattern matching functions were replaced. Previously, commands with special LabVIEW characters could not be executed.\n- Replaced write to file function with write to text file.\n- Replaced while loop with for loop.\n- Replaced 4155C \"Save File\" function and now the vi can save time-dependent variables.\n- Added clock with start time control and various units.\n- Changed filepath in which the program is saved.\n- Added a serial output log that keeps a history.\n- Tab control.\n- Added option for plotting transfer and output curve extrema vs time.\n- Corrected bug of \"itime\" command. The command did not allow for settting the integration time value, it allowed to set the category of the integration time (short, medium, long). If the time value was beyond the range of the category, then the SPA used the closest value allowed, whilst staying in the category. So, if the integration time was changed to long, but the integration time value was a short one, then the SPA would measure using the minimum long integration time value and not the value that the user intended.\n- Added SMU4 command.\n- Added plotting of \"sample\" plots.\n- Added SMU control.\n- Added universal SMU/VSU selector."
  # "Search and replace LF with EOL"
  n1 = Equal?(x="integration time", y=u32 0) -> (x = y?=w59:bool)
  n2 = Select(t="Integration time (short)", s=w59, f="Integration time (long)") -> (s? t:f=w18:dbl)
  n3 = call "4155C Get Filename.vi"("error in (no error)"=errorcluster {"status"=FALSE, "code"=0, "source"=""}) -> ("error out"=w53:errorcluster, "path"=w28:path)  [unwired: 2 in, 1 out]
  "Path" <- w28
  n4 = Bundle By Name(cluster="Timings (overwritten by the Front Panel)", "integration time"="integration time", "Short/Long integration time"=w18) -> (w51:T4)
  n5 = Path To String(path=w28) -> (string=w29:string)
  n6 = Match Pattern(string=w29, regular expression=".txt") -> (before substring=w16:string)  [unwired: 1 in, 3 out]
  n7 = Search and Replace String(replace all?=TRUE ("replace all? (F)"), input string="Script", search string="\n", replace string="\r\n") -> (result string=w41:string)  [unwired: 4 in, 3 out]
  n8 = call "4155C Initialise.vi"("VISA resource name in"="VISA resource name in", "Reset"="Full Reset", "Type of reset"=w58, "error in (no error)"=w53, "VISA Timeout Value"=u32 10000) -> ("VISA Resource Name out"=w52:refnum<visa-resource-name>, "error out"=w8:errorcluster)
  n9 = Concatenate Strings(w16, "-script.txt" ("string")) -> (w17:string)
  n10 = String To Path(string=w17) -> (path=w6:path)
  n11 = Spreadsheet String To Array(delimiter (Tab)="\r\n", format string="%s", spreadsheet string="Script", array type (2D Dbl)="") -> (array=w32:string[][])
  n12 = Open/Create/Replace File(file path (use dialog)=w6, error in=w8, operation (0:open)=T8."replace or create with confirmation") -> (refnum out=w5:refnum<file>, error out=w7:errorcluster)  [unwired: 3 in, 1 out]
  n13 = Array Size(array=w32) -> (size(s)=w36:i32[])
  n14 = Initialize Array("") -> (w22:string[])  [unwired: 1 in]
  n15 = Initialize Array("") -> (w20:string[][])  [unwired: 2 in]
  n16 = Initialize Array(0.0 ("element")) -> (w1:dbl[])  [unwired: 1 in]
  n17 = Index Array(array=w36, index=0) -> (element=w34:i32)
  n18 = Write to Text File(file (use dialog)=w5, text=w41, error in=w7) -> (error out=w25:errorcluster)  [unwired: 1 in, 2 out]
  n19 = for {
    N: w34 -> [w159]
    shift-left: "Source/Drain Range" -> [w199]
    shift-right: [w195] -> _
    shift-left: "Source/Drain\nRange mode" -> [w200]
    shift-right: [w196] -> _
    shift-left: "Gate Range" -> [w201]
    shift-right: [w197] -> _
    shift-left: "Gate Range\nmode" -> [w202]
    shift-right: [w198] -> _
    shift-left: "Gate: Compliance" -> [w211]
    shift-right: [w207] -> _
    shift-left: "Drain: Compliance" -> [w212]
    shift-right: [w208] -> _
    shift-left: w51 -> [w213]
    shift-right: [w209] -> w19
    shift-left: w25 -> [w214]
    shift-right: [w71] -> w27
    shift-left: w52 -> [w215]
    shift-right: [w210] -> _
    shift-left: w16 -> [w216]
    shift-right: [w70] -> _
    tunnel: "Panel Controls 2" -> [w193]
    shift-right: [w112] -> _
    shift-left: w1 -> [w192]
    shift-right: [w146] -> _
    shift-left: i32[] [] -> [w188]
    tunnel: w32 -> [w187] mode=indexing
    shift-right: [w111] -> _
    shift-left: w1 -> [w164]
    shift-right: [w141] -> _
    shift-left: w22 -> [w151]
    shift-right: [w142] -> _
    shift-left: w20 -> [w144]
    shift-right: [w105] -> _
    shift-left: w1 -> [w133]
    shift-right: [w106] -> _
    shift-left: w1 -> [w132]
    shift-right: [w110] -> _
    shift-left: w1 -> [w121]
    shift-right: [w109] -> _
    shift-left: w1 -> [w120]
    shift-right: [w103] -> _
    shift-left: w1 -> [w119]
    shift-right: [w113] -> _
    shift-left: w1 -> [w118]
    shift-right: [w104] -> _
    shift-left: w1 -> [w117]
    shift-right: [w102] -> _
    shift-left: w1 -> [w116]
    shift-right: [w108] -> _
    shift-left: w1 -> [w115]
    shift-right: [w107] -> _
    shift-left: w1 -> [w114]
    shift-right: [w95] -> w3
    shift-left: "Probe 4" -> [w194]
    shift-right: [w66] -> _
    shift-left: w1 -> [w92]
    shift-right: [w67] -> _
    shift-left: w1 -> [w91]
    shift-right: [w68] -> _
    shift-left: w1 -> [w90]
    shift-right: [w69] -> _
    shift-left: w1 -> [w89]
    i -> [w154]
    stop <- "Interrupt program" stop-if-true
    # "Ig for bias stress plots"
    # "Id for bias stress plots"
    # "Is for bias stress plots"
    # "Time axis for bias stress plots"
    # "Save bias stress curves in file."
    # "Is off"
    # "Is on"
    # "Ig off"
    # "Ig on"
    # "Is min"
    # "Is max"
    # "Ig min"
    # "Ig max"
    # "Id min"
    # "Id max"
    # "Id off"
    # "Id on"
    # "Is off"
    # "Is on"
    # "Ig off"
    # "Ig on"
    # "Is min"
    # "Is max"
    # "Ig min"
    # "Ig max"
    # "Id min"
    # "Id max"
    # "Id off"
    # "Id on"
    # "Filepath and name"
    # "Limit of command arguments (array columns). Raise if needed."
    # "Serial port data (string)"
    # "Serial port data (table)"
    # "Serial port data"
    # "For loop counter"
    # "<-----Equivalent to the 4155C \"Write\" subvi.----->"
    # "Headers"
    # "Save transfer curves in file."
    # "Filepath and name"
    # "Save time-dependent data."
    # "Use the time offset if your measurements do not start at t=0."
    # "Time for Imax, Imin, Ion, Ioff"
    # "Rest of elements of command"
    # "First element of command\n(case select)"
    n20 = Add(x=w154, y=1) -> (x+y=→"Line running":i32)
    n21 = Add(x=w159, y=1) -> (x+y=→"Total lines":i32)
    n22 = Index Array(array=w187, index=0 ("line index")) -> (element=w182:string)
    "Command running:" <- w182
    n23 = control-ref of="Interrupt scan"() -> (w206:refnum<vi>)
    n24 = Spreadsheet String To Array(delimiter (Tab)=" ", format string="%s", spreadsheet string=w182, array type (2D Dbl)=string[] []) -> (array=w180:string[])
    n25 = Delete From Array(array=w180, index=0) -> (deleted portion=w134:string, array with subset deleted=w179:string[])  [unwired: 1 in]
    n26 = call "Elapsed Time"("Reset"="Reset", "Auto Reset"="Auto Reset") -> ("Elapsed Time (s)"=w189:dbl)  [unwired: 10 in, 7 out]
    n27 = case shown="2" "Time Units" {
      tunnel: ["-sec" "-min" "-h"] -> w190
      tunnel: [w220 w224 w227] -> w160
      tunnel: w189 -> [w220 w223 w228]
      frame 0, Default {
      }
      frame 1 {
        n28 = Divide(x=w223, y=60.0) -> (x/y=w224:dbl)
      }
      frame 2 {
        n29 = Divide(x=w228, y=3600.0) -> (x/y=w227:dbl)
      }
    }
    n30 = Add(x=w160, y="Time Offset") -> (x+y=w93:dbl)
    n31 = To Long Integer(number=w93) -> (32bit integer=w94:i32)
    "Elapsed Time" <- w94
    n32 = case shown="\"sample\"" w134 {
      tunnel: w179 -> [w264 w301 w337 w353 w479 w596 w740 w864 w1029 w1061 w1134 w1179 w1222 w1261 w1293 _ _ w1479 w1611 _ w1715 w1779 w1840 w1933 w2013 w2051]
      tunnel: w216 -> [w259 w297 w335 w366 w486 w655 w748 w871 w1037 w1078 w1123 w1171 w1215 w1255 w1286 w1323 w1383 w1460 w1593 w1642 w1702 w1766 w1828 w1927 w2009 w2053]
      tunnel: w215 -> [w258 w296 w326 w365 w457 w640 w717 w842 w1005 w1079 w1124 w1172 w1216 w1256 w1287 w1328 w1385 w1485 w1617 w1646 w1721 w1785 w1846 w1939 w1967 w2057]
      tunnel: w214 -> [w257 w295 w325 w364 w456 w639 w716 w841 w1002 w1080 w1125 w1173 w1217 w1257 w1288 w1327 w1356 w1484 w1616 w1645 w1720 w1784 w1845 w1938 w1966 w2056]
      tunnel: w213 -> [w256 w294 w334 w362 w482 w616 w744 w867 w1033 w1088 w1133 w1170 w1214 w1254 w1285 w1326 w1380 w1452 w1585 w1651 w1695 w1759 w1821 w1926 w2008 w2058]
      tunnel: w212 -> [w255 w293 w333 w361 w484 w653 w746 w869 w1035 w1087 w1132 w1178 w1221 w1260 w1292 w1325 w1365 w1483 w1615 w1654 w1719 w1783 w1844 w1937 w2017 w2059]
      tunnel: w211 -> [w254 w292 w332 w359 w483 w652 w745 w868 w1034 w1086 w1131 w1177 w1220 w1259 w1291 w1324 w1366 w1461 w1594 w1653 w1703 w1767 w1829 w1928 w2010 w2061]
      tunnel: [w258 w296 w324 w365 w481 w650 w742 w866 w1031 w1079 w1124 w1172 w1216 w1256 w1287 w1328 w1385 w1453 w1567 w1644 w1696 w1760 w1822 w1880 w1969 w2057] -> w210
      tunnel: [w257 w295 w323 w364 w480 w649 w741 w865 w1030 w1080 w1125 w1173 w1217 w1257 w1288 w1327 w1355 w1462 w1568 w1643 w1704 w1768 w1830 w1879 w1968 w2055] -> w145
      tunnel: [w256 w294 w334 w362 w482 w612 w744 w867 w1033 w1081 w1126 w1170 w1214 w1254 w1285 w1326 w1380 w1452 w1585 w1651 w1695 w1759 w1821 w1926 w2008 w2058] -> w209
      tunnel: [w255 w293 w333 w361 w484 w653 w746 w869 w1035 w1087 w1132 w1178 w1221 w1260 w1292 w1325 w1365 w1483 w1615 w1654 w1719 w1783 w1844 w1937 w2017 w2059] -> w208
      tunnel: [w254 w292 w332 w359 w483 w652 w745 w868 w1034 w1086 w1131 w1177 w1220 w1259 w1291 w1324 w1366 w1461 w1594 w1653 w1703 w1767 w1829 w1928 w2010 w2061] -> w207
      tunnel: [w259 w297 w335 w366 w486 w655 w748 w871 w1037 w1078 w1123 w1171 w1215 w1255 w1286 w1323 w1383 w1460 w1593 w1642 w1702 w1766 w1828 w1927 w2009 w2053] -> w70
      tunnel: w206 -> [_ _ _ _ w488 w659 w753 w873 w1041 _ _ _ _ _ _ _ _ w1457 w1590 _ w1701 w1765 w1827 w1899 w1985 _]
      tunnel: "Gate" -> [_ _ _ _ w466 w643 w727 w851 w1016 _ _ _ _ _ _ _ _ _ _ _ _ _ _ _ _ _]
      tunnel: "Drain 2" -> [_ _ _ _ w465 w642 w726 w850 w1015 _ _ _ _ _ _ _ _ _ _ _ _ _ _ _ _ _]
      tunnel: "Panel Controls" -> [_ _ _ _ _ _ w725 w777 w1014 _ _ _ _ _ _ _ _ _ _ _ _ _ _ _ _ _]
      tunnel: w202 -> [w253 w291 w331 w358 w450 w633 w710 w835 w1000 w1085 w1130 _ w1213 w1253 w1284 w1322 w1367 w1448 w1581 w1647 w1691 w1755 w1817 w1922 w2004 w2062]
      tunnel: w201 -> [w252 w290 w330 w357 w449 w632 w709 w834 w999 w1084 w1129 w1176 _ w1244 w1290 w1321 w1368 w1449 w1582 w1648 w1692 w1756 w1818 w1923 w2005 w2063]
      tunnel: w200 -> [w251 w289 w329 w356 w448 w631 w708 w833 w998 w1083 w1128 w1175 w1219 w1258 _ w1320 w1369 w1450 w1583 w1649 w1693 w1757 w1819 w1924 w2006 w2064]
      tunnel: w199 -> [w250 w288 w328 w355 w447 w630 w707 w832 w1001 w1082 w1127 w1174 w1218 _ w1289 w1319 w1370 w1451 w1584 w1650 w1694 w1758 w1820 w1925 w2007 w2065]
      tunnel: [w253 w291 w331 w358 w450 w633 w710 w835 w1000 w1085 w1130 w1169 w1213 w1253 w1284 w1322 w1367 w1448 w1581 w1647 w1691 w1755 w1817 w1922 w2004 w2062] -> w198
      tunnel: [w252 w290 w330 w357 w449 w632 w709 w834 w999 w1084 w1129 w1176 w1205 w1244 w1290 w1321 w1368 w1449 w1582 w1648 w1692 w1756 w1818 w1923 w2005 w2063] -> w197
      tunnel: [w251 w289 w329 w356 w448 w631 w708 w833 w998 w1083 w1128 w1175 w1219 w1258 w1283 w1320 w1369 w1450 w1583 w1649 w1693 w1757 w1819 w1924 w2006 w2064] -> w196
      tunnel: [w250 w288 w328 w355 w447 w630 w707 w832 w1001 w1082 w1127 w1174 w1218 w1245 w1289 w1319 w1370 w1451 w1584 w1650 w1694 w1758 w1820 w1925 w2007 w2065] -> w195
      tunnel: w194 -> [w234 w269 w306 _ w388 w585 w679 w773 w969 w1058 w1106 w1153 w1189 w1228 w1267 w1303 w1333 w1435 w1547 w1626 w1662 w1730 w1793 w1859 w1944 w2022]
      tunnel: w193 -> [_ _ _ _ w441 w627 _ _ _ _ _ _ _ _ _ _ _ _ _ _ _ _ _ _ _ _]
      tunnel: [w249 w284 w321 w370 w403 w604 w697 w789 w987 w1077 w1121 w1168 w1204 w1243 w1282 w1318 w1351 w1425 w1551 w1641 w1680 w1748 w1811 w1877 w1962 w2054] -> w112
      tunnel: w192 -> [w249 w284 w321 w370 w438 w604 w697 w824 w987 w1077 w1121 w1168 w1204 w1243 w1282 w1318 w1351 w1431 w1551 w1641 w1680 w1748 w1811 w1877 w1962 w2054]
      tunnel: w93 -> [_ _ _ _ w437 w601 w695 w823 w984 _ _ _ _ _ _ _ w1349 w1440 w1563 _ w1677 w1745 w1808 w1874 w1958 _]
      tunnel: w190 -> [_ _ _ _ w434 w600 w693 w820 w983 _ _ _ _ _ _ _ w1347 w1438 w1562 _ w1676 w1744 w1807 w1873 w1959 _]
      tunnel: w94 -> [_ _ _ _ w430 _ _ w816 _ _ _ _ _ _ _ _ _ _ _ _ _ _ _ _ _ _]
      tunnel: [w248 w283 w320 w360 w407 w603 w696 w793 w986 w1076 w1120 w1167 w1203 w1242 w1281 w1317 w1350 w1410 w1565 w1640 w1679 w1747 w1810 w1876 w1961 w2060] -> w146
      tunnel: w188 -> [w248 w283 w320 w360 w433 w603 w696 w819 w986 w1076 w1120 w1167 w1203 w1242 w1281 w1317 w1350 w1412 w1565 w1640 w1679 w1747 w1810 w1876 w1961 w2060]
      tunnel: [w247 w282 w319 w369 w402 w599 w692 w788 w982 w1075 w1119 w1166 w1202 w1241 w1280 w1316 w1346 w1424 w1550 w1639 w1675 w1743 w1806 w1872 w1957 w2049] -> w111
      tunnel: w164 -> [w247 w282 w319 w369 w429 w599 w692 w815 w982 w1075 w1119 w1166 w1202 w1241 w1280 w1316 w1346 w1430 w1550 w1639 w1675 w1743 w1806 w1872 w1957 w2049]
      tunnel: [w246 w281 w318 w354 w422 w598 w691 w808 w981 w1074 w1118 w1165 w1201 w1240 w1279 w1315 w1345 w1437 w1561 w1638 w1674 w1742 w1805 w1871 w1956 w2048] -> w141
      tunnel: w151 -> [w246 w281 w318 w354 w422 w598 w691 w808 w981 w1074 w1118 w1165 w1201 w1240 w1279 w1315 w1345 w1437 w1561 w1638 w1674 w1742 w1805 w1871 w1956 w2047]
      tunnel: [w245 w280 w317 w363 w421 w597 w690 w807 w980 w1073 w1117 w1164 w1200 w1239 w1278 w1314 w1344 w1436 w1560 w1637 w1673 w1741 w1804 w1870 w1955 w2033] -> w142
      tunnel: w144 -> [w245 w280 w317 w363 w421 w597 w690 w807 w980 w1073 w1117 w1164 w1200 w1239 w1278 w1314 w1344 w1436 w1560 w1637 w1673 w1741 w1804 w1870 w1955 w2033]
      tunnel: [w243 w278 w315 w375 w396 w594 w688 w782 w978 w1071 w1116 w1163 w1198 w1237 w1276 w1312 w1342 w1418 w1559 w1636 w1672 w1740 w1802 w1869 w1954 w2032] -> w105
      tunnel: w133 -> [w243 w278 w315 w375 w420 w594 w688 w806 w978 w1071 w1116 w1163 w1198 w1237 w1276 w1312 w1342 w1418 w1559 w1636 w1672 w1740 w1802 w1869 w1954 w2032]
      tunnel: [w244 w279 w316 w376 w397 w595 w689 w783 w979 w1072 w1115 w1162 w1199 w1238 w1277 w1313 w1343 w1419 w1558 w1635 w1671 w1739 w1803 w1868 w1953 w2031] -> w106
      tunnel: w132 -> [w244 w279 w316 w376 w419 w595 w689 w805 w979 w1072 w1115 w1162 w1199 w1238 w1277 w1313 w1343 w1419 w1558 w1635 w1671 w1739 w1803 w1868 w1953 w2031]
      tunnel: [w236 w271 w308 w368 w401 w591 w686 w787 w976 w1064 w1113 w1160 w1196 w1235 w1274 w1310 w1335 w1423 w1549 w1634 w1664 w1732 w1795 w1861 w1948 w2024] -> w110
      tunnel: w121 -> [w236 w271 w308 w368 w415 w591 w686 w801 w976 w1064 w1113 w1160 w1196 w1235 w1274 w1310 w1335 w1429 w1549 w1634 w1664 w1732 w1795 w1861 w1948 w2024]
      tunnel: [w235 w270 w307 w367 w400 w592 w687 w786 w977 w1063 w1114 w1161 w1197 w1236 w1275 w1311 w1334 w1422 w1548 w1633 w1663 w1731 w1794 w1860 w1947 w2023] -> w109
      tunnel: w120 -> [w235 w270 w307 w367 w414 w592 w687 w800 w977 w1063 w1114 w1161 w1197 w1236 w1275 w1311 w1334 w1428 w1548 w1633 w1663 w1731 w1794 w1860 w1947 w2023]
      tunnel: [w238 w273 w310 w372 w406 w590 w684 w792 w974 w1069 w1111 w1158 w1194 w1233 w1272 w1308 w1337 w1427 w1553 w1628 w1666 w1734 w1797 w1863 w1946 w2028] -> w103
      tunnel: w119 -> [w238 w273 w310 w372 w413 w590 w684 w799 w974 w1069 w1111 w1158 w1194 w1233 w1272 w1308 w1337 w1433 w1553 w1628 w1666 w1734 w1797 w1863 w1946 w2028]
      tunnel: [w237 w272 w309 w371 w404 w593 w685 w790 w975 w1070 w1112 w1159 w1195 w1234 w1273 w1309 w1336 w1426 w1552 w1627 w1665 w1733 w1796 w1862 w1945 w2027] -> w113
      tunnel: w118 -> [w237 w272 w309 w371 w412 w593 w685 w798 w975 w1070 w1112 w1159 w1195 w1234 w1273 w1309 w1336 w1432 w1552 w1627 w1665 w1733 w1796 w1862 w1945 w2027]
      tunnel: [w240 w275 w312 w374 w395 w589 w682 w781 w972 w1067 w1109 w1156 w1192 w1231 w1270 w1306 w1339 w1417 w1555 w1630 w1668 w1736 w1799 w1865 w1950 w2030] -> w104
      tunnel: w117 -> [w240 w275 w312 w374 w411 w589 w682 w797 w972 w1067 w1109 w1156 w1192 w1231 w1270 w1306 w1339 w1417 w1555 w1630 w1668 w1736 w1799 w1865 w1950 w2030]
      tunnel: [w239 w274 w311 w373 w394 w588 w683 w780 w973 w1068 w1110 w1157 w1193 w1232 w1271 w1307 w1338 w1416 w1554 w1629 w1667 w1735 w1798 w1864 w1949 w2029] -> w102
      tunnel: w116 -> [w239 w274 w311 w373 w410 w588 w683 w796 w973 w1068 w1110 w1157 w1193 w1232 w1271 w1307 w1338 w1416 w1554 w1629 w1667 w1735 w1798 w1864 w1949 w2029]
      tunnel: [w242 w277 w314 w378 w399 w587 w680 w785 w970 w1065 w1107 w1154 w1190 w1229 w1268 w1304 w1341 w1421 w1557 w1632 w1670 w1738 w1801 w1867 w1952 w2026] -> w108
      tunnel: w115 -> [w242 w277 w314 w378 w409 w587 w680 w795 w970 w1065 w1107 w1154 w1190 w1229 w1268 w1304 w1341 w1421 w1557 w1632 w1670 w1738 w1801 w1867 w1952 w2026]
      tunnel: [w241 w276 w313 w377 w398 w586 w681 w784 w971 w1066 w1108 w1155 w1191 w1230 w1269 w1305 w1340 w1420 w1556 w1631 w1669 w1737 w1800 w1866 w1951 w2025] -> w107
      tunnel: w114 -> [w241 w276 w313 w377 w408 w586 w681 w794 w971 w1066 w1108 w1155 w1191 w1230 w1269 w1305 w1340 w1420 w1556 w1631 w1669 w1737 w1800 w1866 w1951 w2025]
      tunnel: [w234 w269 w306 w344 w388 w585 w679 w773 w969 w1058 w1106 w1153 w1189 w1228 w1267 w1303 w1333 w1435 w1547 w1626 w1662 w1730 w1793 w1859 w1944 w2022] -> w95
      tunnel: w93 -> [_ _ _ _ _ _ _ _ _ _ _ _ _ _ _ _ _ w1387 _ _ _ _ _ _ _ _]
      tunnel: [w233 w268 w305 w343 w387 w584 w678 w772 w968 w1057 w1105 w1152 w1188 w1227 w1266 w1302 w1332 w1399 w1546 w1625 w1661 w1729 w1792 w1858 w1943 w2021] -> w66
      tunnel: [w232 w267 w304 w342 w386 w583 w677 w771 w967 w1056 w1104 w1151 w1187 w1226 w1265 w1301 w1331 w1396 w1545 w1624 w1660 w1728 w1791 w1857 w1942 w2020] -> w67
      tunnel: [w231 w266 w303 w341 w385 w582 w676 w770 w966 w1055 w1103 w1150 w1186 w1225 w1264 w1300 w1330 w1397 w1544 w1623 w1659 w1727 w1790 w1856 w1941 w2019] -> w68
      tunnel: [w230 w265 w302 w340 w384 w581 w675 w769 w965 w1054 w1102 w1149 w1185 w1224 w1263 w1299 w1329 w1398 w1543 w1622 w1658 w1726 w1789 w1855 w1940 w2018] -> w69
      tunnel: w92 -> [w233 w268 w305 w343 w387 w584 w678 w772 w968 w1057 w1105 w1152 w1188 w1227 w1266 w1302 w1332 w1403 w1546 w1625 w1661 w1729 w1792 w1858 w1943 w2021]
      tunnel: w91 -> [w232 w267 w304 w342 w386 w583 w677 w771 w967 w1056 w1104 w1151 w1187 w1226 w1265 w1301 w1331 w1402 w1545 w1624 w1660 w1728 w1791 w1857 w1942 w2020]
      tunnel: w90 -> [w231 w266 w303 w341 w385 w582 w676 w770 w966 w1055 w1103 w1150 w1186 w1225 w1264 w1300 w1330 w1401 w1544 w1623 w1659 w1727 w1790 w1856 w1941 w2019]
      tunnel: w89 -> [w230 w265 w302 w340 w384 w581 w675 w769 w965 w1054 w1102 w1149 w1185 w1224 w1263 w1299 w1329 w1400 w1543 w1622 w1658 w1726 w1789 w1855 w1940 w2018]
      tunnel: "Standby" -> [_ _ _ _ w383 w580 _ w768 _ _ _ _ _ _ _ _ _ w1394 w1542 _ _ _ _ w1854 _ _]
      frame "wait" {
        n33 = Index Array(array=w264, index=0 ("Index")) -> (element=w262:string)
        n34 = Decimal String To Number(string=w262, default (0L)=u32 0) -> (number=w261:u32)  [unwired: 1 in, 1 out]
        n35 = Wait (ms)(milliseconds to wait=w261) -> ()  [unwired: 1 out]
      }
      frame "wait-min" {
        n36 = Index Array(array=w301, index=0 ("Index")) -> (element=w299:string)
        n37 = Decimal String To Number(string=w299, default (0L)=u32 0) -> (number=w287:u32)  [unwired: 1 in, 1 out]
        n38 = Multiply(x=w287, y=u32 60000) -> (x*y=w286:u32)
        n39 = Wait (ms)(milliseconds to wait=w286) -> ()  [unwired: 1 out]
      }
      frame "standby" {
        n40 = Index Array(array=w337, index=0 ("Index")) -> (element=w327:string)
        n41 = case shown="\"off\", Default" w327 {
          tunnel: [":PAGE:SCON:STAN 0" ":PAGE:SCON:STAN 1"] -> w322
          frame "off", Default {
          }
          frame "on" {
          }
        }
        n42 = VISA Write(VISA resource name=w326, write buffer=w322, error in (no error)=w325) -> (VISA resource name out=w324:refnum<visa-resource-name>, error out=w323:errorcluster)  [unwired: 1 out]
      }
      frame "Probe4" {
        n43 = Delete From Array(array=w353, index=0) -> (deleted portion=w347:string, array with subset deleted=w350:string[])  [unwired: 1 in]
        n44 = Equal?(x=w347, y="ON") -> (x = y?=w345:bool)
        n45 = Delete From Array(array=w350, index=0) -> (deleted portion=w349:string)  [unwired: 1 in, 1 out]
        n46 = Fract/Exp String To Number(string=w349) -> (number=w346:dbl)  [unwired: 3 in, 1 out]
        n47 = Bundle(w345, w346) -> (w344:cluster{bool, dbl})  [unwired: 1 in]
      }
      frame "transfer" {
        n48 = local read "Transfer/Output - Gate"() -> (w382:u32)
        n49 = Delete From Array(array=w479, index=0 ("Index")) -> (deleted portion=w477:string, array with subset deleted=w476:string[])  [unwired: 1 in]
        n50 = Bundle By Name(cluster=w441, "Emergency Stop"=w488) -> (w442:T2)
        n51 = Number To Decimal String(number=w437) -> (decimal integer string=w436:string)  [unwired: 1 in]
        n52 = case shown="\"d\", Default" w477 {
          tunnel: [w573 w574] -> w475
          frame "s" {
            w573 = u16 0 items=["Single", "Double"] ("sweep mode")
          }
          frame "d", Default {
            w574 = u16 1 items=["Single", "Double"] ("sweep mode")
          }
        }
        n53 = Fract/Exp String To Number(string=w476) -> (number=w461:dbl[])  [unwired: 3 in, 1 out]
        n54 = Concatenate Strings(w486, "-transfer-" ("Prefix"), w436, w434, ".txt" ("Suffix (transfer)")) -> (w487:string)
        n55 = VISA Write(VISA resource name=w457, write buffer=":PAGE:CHAN:MODE SWE;" ("write buffer (\"\")"), error in (no error)=w456) -> (VISA resource name out=w454:refnum<visa-resource-name>, error out=w455:errorcluster)  [unwired: 1 out]
        n56 = local read "Plot transfer curve extrema vs time"() -> (w389:bool)
        n57 = String To Path(string=w487) -> (path=w485:path)
        n58 = Index Array(array=w461, index #1=0 ("Index")) -> (element #1=w474:dbl, element #2=w473:dbl, element #3=w472:dbl)  [unwired: 2 in]
        n59 = Delete From Array(array=w461, length=3 ("Length"), index=0 ("Index")) -> (array with subset deleted=w459:dbl[])  [unwired: 1 out]
        n60 = local read "Transfer/Output - Drain"() -> (w379:u32)
        n61 = local read "Transfer/Output - Source/Common"() -> (w381:u32)
        n62 = case shown="True" w389 {
          tunnel: w433 -> [w490 w493]
          tunnel: w430 -> [_ w492]
          tunnel: [w490 w491] -> w407
          frame False {
          }
          frame True {
            n63 = Build Array (concatenate)(w493, w492) -> (w491:i32[])
          }
        }
        n64 = local read "Transfer/Output - Probe 4"() -> (w380:u32)
        n65 = Bundle By Name(cluster=w466, "Gate Start"=w474, "Gate Stop"=w473, "Gate Step (linear only)"=w472, "Gate Compliance"=w483, "Range mode"=w450, "Range"=w449) -> (w451:T6)
        n66 = Index Array(array=w459, index #1=0 ("Index")) -> (element #1=w469:dbl, element #2=w468:dbl, element #3=w467:dbl)  [unwired: 2 in]
        n67 = call <vilib>:"compatOverwrite.vi"("overwrite (F)"=TRUE) -> ("overwrite?"=w440:T8)
        n68 = Bundle By Name(cluster=w465, "Drain Start"=w469, "Drain Stop"=w468, "Drain Step"=w467, "Drain Compliance"=w484, "Range mode"=w448, "Range"=w447) -> (w452:T7)
        n69 = call "4155C Transfer v3.0.vi"("VISA resource name in"=w454, "Source/Common"=w381, 2:"Gate"=w451, 3:"Drain"=w452, 4:"Drain"=w379, "Timings"=w482, "error in (no error)"=w455, 7:"Probe 4"=w388, 8:"Gate"=w382, 9:"Probe 4"=w380, "sweep mode"=w475, "Panel Controls"=w442, "Standby"=w383) -> ("VG"=w439:dbl[], "Outparams"=w446:T9, "VISA Resource Name out"=w481:refnum<visa-resource-name>, "IS"=w417:dbl[], "ID"=w418:dbl[], "IG"=w416:dbl[], "error out"=w431:errorcluster, "Probe 4"=w443:dbl[])  [unwired: 7 in]
        n70 = Unbundle By Name(w446) -> ("V2 Step"=w445:dbl, "V2 Start"=w444:dbl, "Number of points"=w405:i32)
        n71 = call "4155C Split array.vi"("Number of VAR2 steps"=w405, "Y2 data in"=w418, "X data in"=w439, "Y1 data in"=w417, "Y3 data in"=w416, "error in (no error)"=w431) -> ("Array of clusters"=w432:cluster{"Y data in":dbl[], "X data in":dbl[]}[], "error out"=w393:errorcluster)  [unwired: 1 in]
        n72 = case shown="True" "Plot transfer curve extrema vs time" {
          tunnel: w438 -> [w496 w572]
          tunnel: w429 -> [w497 w567]
          tunnel: w420 -> [w503 w563]
          tunnel: w419 -> [w504 w562]
          tunnel: w418 -> [_ w559]
          tunnel: w417 -> [_ w557]
          tunnel: w416 -> [_ w556]
          tunnel: w415 -> [w498 w552]
          tunnel: w414 -> [w500 w551]
          tunnel: w413 -> [w494 w548]
          tunnel: w412 -> [w495 w547]
          tunnel: w411 -> [w502 w544]
          tunnel: w410 -> [w501 w543]
          tunnel: w409 -> [w506 w540]
          tunnel: w408 -> [w505 w539]
          tunnel: w407 -> [_ w532]
          tunnel: [w494 w527] -> w406
          tunnel: w405 -> [_ w526]
          tunnel: [w495 w525] -> w404
          tunnel: [w496 w524] -> w403
          tunnel: [w497 w523] -> w402
          tunnel: [w498 w522] -> w401
          tunnel: [w500 w521] -> w400
          tunnel: [w506 w520] -> w399
          tunnel: [w505 w519] -> w398
          tunnel: [w504 w518] -> w397
          tunnel: [w503 w517] -> w396
          tunnel: [w502 w516] -> w395
          tunnel: [w501 w515] -> w394
          tunnel: w393 -> [w499 w514]
          tunnel: [w499 w510] -> w392
          frame False {
          }
          frame True {
            # "Adjusts graph colors."
            # "Adjusts graph colors."
            # "Ion will be the middle element of the array. The calculation of the index is done only once, since Is, Id, and Ig have the same dimensions."
            # "abs(Ig)"
            # "abs(Is)"
            # "Y1: Is\nY2: Id\nY3: Ig"
            # "abs(Id)"
            # "Adjusts graph colors."
            # "Adjusts graph colors."
            # "Adjusts graph colors."
            n73 = Absolute Value(x=w557) -> (abs(x)=w542:dbl[])
            n74 = Absolute Value(x=w559) -> (abs(x)=w558:dbl[])
            n75 = Absolute Value(x=w556) -> (abs(x)=w545:dbl[])
            n76 = Array Size(array=w558) -> (size(s)=w566:i32)
            n77 = Divide(x=w566, y=2) -> (x/y=w509:dbl)
            n78 = Subtract(x=w509, y=1) -> (x-y=w508:dbl)
            n79 = Array Max & Min(array=w542) -> (max value=w549:dbl, min value=w550:dbl)  [unwired: 2 out]
            n80 = Array Max & Min(array=w558) -> (max value=w571:dbl, min value=w555:dbl)  [unwired: 2 out]
            n81 = Array Max & Min(array=w545) -> (max value=w554:dbl, min value=w553:dbl)  [unwired: 2 out]
            n82 = Index Array(array=w542, index=w508) -> (element=w533:dbl)
            n83 = Index Array(array=w542, index=0) -> (element=w534:dbl)
            n84 = Index Array(array=w558, index=w508) -> (element=w535:dbl)
            n85 = Index Array(array=w558, index=0) -> (element=w536:dbl)
            n86 = Index Array(array=w545, index=w508) -> (element=w538:dbl)
            n87 = Index Array(array=w545, index=0) -> (element=w537:dbl)
            n88 = local write "Ig max"(w554) -> ()
            n89 = local write "Ig min"(w553) -> ()
            n90 = local write "Is max"(w549) -> ()
            n91 = local write "Is min"(w550) -> ()
            n92 = local write "Id max"(w571) -> ()
            n93 = local write "Id min"(w555) -> ()
            n94 = Build Array (concatenate)(w548, w549) -> (w527:dbl[])
            n95 = Build Array (concatenate)(w547, w550) -> (w525:dbl[])
            n96 = local write "Is off"(w534) -> ()
            n97 = local write "Is on"(w533) -> ()
            n98 = Build Array (concatenate)(w572, w571) -> (w524:dbl[])
            n99 = Build Array (concatenate)(w567, w555) -> (w523:dbl[])
            n100 = Build Array (concatenate)(w552, w554) -> (w522:dbl[])
            n101 = Build Array (concatenate)(w551, w553) -> (w521:dbl[])
            n102 = Build Array (concatenate)(w540, w533) -> (w520:dbl[])
            n103 = Build Array (concatenate)(w539, w534) -> (w519:dbl[])
            n104 = Build Array (concatenate)(w562, w535) -> (w518:dbl[])
            n105 = Build Array (concatenate)(w563, w536) -> (w517:dbl[])
            n106 = Build Array (concatenate)(w544, w538) -> (w516:dbl[])
            n107 = Build Array (concatenate)(w543, w537) -> (w515:dbl[])
            n108 = local write "Ig off"(w537) -> ()
            n109 = local write "Ig on"(w538) -> ()
            n110 = local write "Id off"(w536) -> ()
            n111 = local write "Id on"(w535) -> ()
            n112 = control-ref of="Imax vs time"() -> (w561:refnum<vi>)
            n113 = control-ref of="Imin vs time"() -> (w560:refnum<vi>)
            n114 = control-ref of="Ion vs time"() -> (w529:refnum<vi>)
            n115 = control-ref of="Ioff vs time"() -> (w528:refnum<vi>)
            n116 = control-ref of="I vs Vg"() -> (w570:refnum<vi>)
            n117 = call "4155C Split array.vi"("Number of VAR2 steps"=w526, "Y2 data in"=w518, "X data in"=w532, "Y1 data in"=w520, "Y3 data in"=w516, "error in (no error)"=w514) -> ("Array of clusters"=w530:cluster{"Y data in":dbl[], "X data in":dbl[]}[], "error out"=w513:errorcluster)  [unwired: 1 in]
            n118 = call "4155C Split array.vi"("Number of VAR2 steps"=w526, "Y2 data in"=w517, "X data in"=w532, "Y1 data in"=w519, "Y3 data in"=w515, "error in (no error)"=w513) -> ("Array of clusters"=w531:cluster{"Y data in":dbl[], "X data in":dbl[]}[], "error out"=w512:errorcluster)  [unwired: 1 in]
            n119 = call "4155C Split array.vi"("Number of VAR2 steps"=w526, "Y2 data in"=w524, "X data in"=w532, "Y1 data in"=w527, "Y3 data in"=w522, "error in (no error)"=w512) -> ("Array of clusters"=w569:cluster{"Y data in":dbl[], "X data in":dbl[]}[], "error out"=w511:errorcluster)  [unwired: 1 in]
            n120 = call "4155C Split array.vi"("Number of VAR2 steps"=w526, "Y2 data in"=w523, "X data in"=w532, "Y1 data in"=w525, "Y3 data in"=w521, "error in (no error)"=w511) -> ("Array of clusters"=w568:cluster{"Y data in":dbl[], "X data in":dbl[]}[], "error out"=w510:errorcluster)  [unwired: 1 in]
            n121 = call "4155C Config Chart Colours.vi"("Numeric"=w526, "XY Graph 2"=w561) -> ()  [unwired: 6 in]
            n122 = call "4155C Config Chart Colours.vi"("Numeric"=w526, "XY Graph 2"=w560) -> ()  [unwired: 6 in]
            n123 = call "4155C Config Chart Colours.vi"("Numeric"=w526, "XY Graph 2"=w529) -> ()  [unwired: 6 in]
            n124 = call "4155C Config Chart Colours.vi"("Numeric"=w526, "XY Graph 2"=w528) -> ()  [unwired: 6 in]
            n125 = call "4155C Config Chart Colours.vi"("Numeric"=w526, "XY Graph 2"=w570) -> ()  [unwired: 6 in]
            n126 = local write "Imax vs time"(w569) -> ()
            n127 = local write "Imin vs time"(w568) -> ()
            n128 = local write "Ion vs time"(w530) -> ()
            n129 = local write "Ioff vs time"(w531) -> ()
          }
        }
        n130 = local write "I vs Vg"(w432) -> ()
        n131 = Open/Create/Replace File(file path (use dialog)=w485, error in=w392, operation (0:open)=w440) -> (refnum out=w427:refnum<file>, error out=w425:errorcluster)  [unwired: 3 in, 1 out]
        n132 = call "4155C Make Big 2d array.vi"("1D Var1"=w439, "1d IS"=w417, "1d ID"=w418, "1d IG"=w416, "1d SMU4"=w443, "SMU4"=w388, "VAR2 START"=w444, "Number of VAR2 steps"=w405, "VAR2 STEP"=w445, "VAR1 Name"="Vg", "Decimal places in header"=i8 1, "VAR2 Name"="Vd") -> ("Header array"=w428:string[], "Data array"=w426:dbl[][])  [unwired: 14 in]
        n133 = call "4155C Write array to file.vi"("Byte Stream File Refnum"=w427, "Header"=w428, "Data Array"=w426, "error in (no error)"=w425) -> ("dup refnum"=w424:refnum<file>, "error out"=w423:errorcluster)  [unwired: 1 in]
        n134 = Close File(refnum=w424, error in=w423) -> (error out=w480:errorcluster)  [unwired: 1 out]
      }
      frame "pulsedstressV" {
        w610 = 0
        n135 = local read "Pulsed Stress V - Drain"() -> (w579:u32)
        n136 = local read "Pulsed Stress V - Gate"() -> (w576:u32)
        n137 = local read "Pulsed Stress V - Probe 4"() -> (w578:u32)
        n138 = local read "Pulsed Stress V - Source/Common"() -> (w575:u32)
        n139 = local read "Pulsed Stress V - Vextra"() -> (w577:u32)
        n140 = Number To Decimal String(number=w601) -> (decimal integer string=w656:string)  [unwired: 1 in]
        n141 = Delete From Array(array=w596, index=0 ("Index")) -> (deleted portion=w647:string, array with subset deleted=w646:string[])  [unwired: 1 in]
        n142 = Bundle By Name(cluster=w627, "Emergency Stop"=w659) -> (w628:T2)
        n143 = VISA Write(VISA resource name=w640, write buffer=":PAGE:CHAN:MODE SWE;" ("write buffer (\"\")"), error in (no error)=w639) -> (VISA resource name out=w637:refnum<visa-resource-name>, error out=w638:errorcluster)  [unwired: 1 out]
        n144 = Concatenate Strings(w655, "-pulsedstressV-" ("Substring"), w656, w600, ".txt" ("Substring")) -> (w658:string)
        n145 = case shown="\"d\", Default" w647 {
          tunnel: [w668 w669] -> w645
          frame "s" {
            w668 = u16 0 items=["Single", "Double"] ("sweep mode")
          }
          frame "d", Default {
            w669 = u16 1 items=["Single", "Double"] ("sweep mode")
          }
        }
        n146 = Fract/Exp String To Number(string=w646) -> (number=w641:dbl[])  [unwired: 3 in, 1 out]
        n147 = String To Path(string=w658) -> (path=w654:path)
        n148 = Index Array(array=w641, index #1=0 ("Index")) -> (element #1=w619:dbl, element #2=w618:dbl, element #3=w615:dbl, element #4=w614:dbl, element #5=w613:dbl, element #6=w617:dbl)  [unwired: 5 in]
        n149 = Bundle By Name(cluster=w616, "Pulse period"=w614, "Base voltage"=w615, "Pulse width"=w613) -> (w612:T4)
        n150 = Unbundle By Name(w612) -> ("Pulse period"=w620:dbl)
        n151 = Bundle By Name(cluster=w643, "Gate Start"=w618, "Gate Stop"=w619, "Gate Step (linear only)"=0, "Gate Compliance"=w652, "Range mode"=w633, "Range"=w632) -> (w634:T6)
        n152 = call <vilib>:"compatOverwrite.vi"("overwrite (F)"=TRUE) -> ("overwrite?"=w605:T8)
        n153 = Bundle By Name(cluster=w642, "Drain Start"=w617, "Drain Stop"=w610, "Drain Step"=w610, "Drain Compliance"=w653, "Range mode"=w631, "Range"=w630) -> (w635:T7)
        n154 = call "4155C PulsedStressV v3.0.vi"("VISA resource name in"=w637, "Gate"=w634, "Pulsed Stress V - Source/Common"=w575, "Drain"=w635, "Timings"=w612, "error in (no error)"=w638, "sweep mode"=w645, "Probe 4"=w585, "Pulsed Stress V - Drain"=w579, "Pulsed Stress V - Gate"=w576, "Panel Controls"=w628, "Standby"=w580, "Pulsed Stress V - Probe 4"=w578, "Pulsed Stress V - Vextra"=w577) -> ("Outparams"=w629:T9, "VISA Resource Name out"=w650:refnum<visa-resource-name>, "ID"=w608:dbl[], "IG"=w606:dbl[], "error out"=w651:errorcluster)  [unwired: 1 in]
        n155 = Unbundle By Name(w629) -> ("Number of points"=w607:i32)  [unwired: 2 out]
        n156 = for {
          N: w607 -> [_]
          tunnel: [w665] -> w609 mode=indexing
          tunnel: w620 -> [w667]
          i -> [w666]
          n157 = Multiply(x=w667, y=w666) -> (x*y=w665:dbl)
        }
        n158 = Insert Into Array(array=dbl[][] [] ("Input Array"), new element=w609) -> (w621:dbl[][])  [unwired: 2 in]
        n159 = Insert Into Array(array=w621, new element=w608) -> (w626:dbl[][])  [unwired: 2 in]
        n160 = Insert Into Array(array=w626, new element=w606) -> (w625:dbl[][])  [unwired: 2 in]
        n161 = Transpose 2D Array(2D array=w625) -> (transposed array=w624:dbl[][])
        n162 = Open/Create/Replace File(file path (use dialog)=w654, error in=w651, operation (0:open)=w605) -> (refnum out=w662:refnum<file>, error out=w663:errorcluster)  [unwired: 3 in, 1 out]
        n163 = call "4155C Write array to file.vi"("Byte Stream File Refnum"=w662, "Header"=string[] ["Time /s", "Id /A", "Ig /A"], "Data Array"=w624, "error in (no error)"=w663) -> ("dup refnum"=w660:refnum<file>, "error out"=w661:errorcluster)  [unwired: 1 in]
        n164 = Close File(refnum=w660, error in=w661) -> (error out=w649:errorcluster)  [unwired: 1 out]
      }
      frame "transfer-fpp" {
        n165 = local read "FPP - Source"() -> (w674:u32)
        n166 = local read "FPP - Drain"() -> (w672:u32)
        n167 = local read "FPP - Gate"() -> (w673:u32)
        n168 = local read "FPP - Probe 1"() -> (w670:u32)
        n169 = local read "FPP - Probe 2"() -> (w671:u32)
        n170 = Number To Decimal String(number=w695) -> (decimal integer string=w749:string)  [unwired: 1 in]
        n171 = Bundle By Name(cluster=w725, "Emergency Stop"=w753) -> (w761:T1)
        n172 = Delete From Array(array=w740, index=0 ("Index")) -> (deleted portion=w738:string, array with subset deleted=w737:string[])  [unwired: 1 in]
        n173 = Concatenate Strings(w748, "-transferfpp-" ("Substring"), w749, w693, ".txt" ("Substring")) -> (w751:string)
        n174 = VISA Write(VISA resource name=w717, write buffer=":PAGE:CHAN:MODE SWE;" ("write buffer (\"\")"), error in (no error)=w716) -> (VISA resource name out=w714:refnum<visa-resource-name>, error out=w715:errorcluster)  [unwired: 1 out]
        n175 = case shown="\"d\", Default" w738 {
          tunnel: [w762 w763] -> w736
          frame "s" {
            w762 = u16 0 items=["Single", "Double"] ("sweep mode")
          }
          frame "d", Default {
            w763 = u16 1 items=["Single", "Double"] ("sweep mode")
          }
        }
        n176 = Fract/Exp String To Number(string=w737) -> (number=w721:dbl[])  [unwired: 3 in, 1 out]
        n177 = String To Path(string=w751) -> (path=w747:path)
        n178 = Index Array(array=w721, index #1=0 ("Index")) -> (element #1=w735:dbl, element #2=w734:dbl, element #3=w733:dbl)  [unwired: 2 in]
        n179 = Delete From Array(array=w721, length=3 ("Length"), index=0 ("Index")) -> (array with subset deleted=w719:dbl[])  [unwired: 1 out]
        n180 = Bundle By Name(cluster=w727, "Gate Start"=w735, "Gate Stop"=w734, "Gate Step (linear only)"=w733, "Gate Compliance"=w745, "Range mode"=w710, "Range"=w709) -> (w711:T6)
        n181 = Index Array(array=w719, index #1=0 ("Index")) -> (element #1=w730:dbl, element #2=w729:dbl, element #3=w728:dbl)  [unwired: 2 in]
        n182 = call <vilib>:"compatOverwrite.vi"("overwrite (F)"=TRUE) -> ("overwrite?"=w698:T8)
        n183 = Bundle By Name(cluster=w726, "Drain Start"=w730, "Drain Stop"=w729, "Drain Step"=w728, "Drain Compliance"=w746, "Range mode"=w708, "Range"=w707) -> (w712:T7)
        n184 = call "4155C Transfer-FPP v3.0.vi"("VISA resource name in"=w714, "FPP - Source"=w674, "Gate"=w711, "Drain"=w712, "FPP - Drain"=w672, "Timings"=w744, "error in (no error)"=w715, "FPP - Gate"=w673, "FPP - Probe 1"=w670, "sweep mode"=w736, "FPP - Probe 2"=w671, "Panel Controls"=w761) -> ("VG"=w752:dbl[], "Outparams"=w706:T9, "VISA Resource Name out"=w742:refnum<visa-resource-name>, "Vprobe2"=w702:dbl[], "ID"=w701:dbl[], "IG"=w700:dbl[], "Vprobe1"=w699:dbl[], "error out"=w743:errorcluster)  [unwired: 8 in]
        n185 = Unbundle By Name(w706) -> ("V2 Step"=w705:dbl, "V2 Start"=w704:dbl, "Number of points"=w703:i32)
        n186 = Open/Create/Replace File(file path (use dialog)=w747, error in=w743, operation (0:open)=w698) -> (refnum out=w758:refnum<file>, error out=w759:errorcluster)  [unwired: 3 in, 1 out]
        n187 = call "4155C Make Big 2d array FPP.vi"("1D Var1"=w752, "1d ID"=w701, "1d Vp2"=w702, "1d IG"=w700, "1d Vp1"=w699, "VAR2 START"=w704, "Number of VAR2 steps"=w703, "VAR2 STEP"=w705, "VAR1 Name"="Vg", "Decimal places in header"=i8 1, "VAR2 Name"="Vd") -> ("Header array"=w754:string[], "Data array"=w755:dbl[][])  [unwired: 15 in]
        n188 = call "4155C Write array to file.vi"("Byte Stream File Refnum"=w758, "Header"=w754, "Data Array"=w755, "error in (no error)"=w759) -> ("dup refnum"=w756:refnum<file>, "error out"=w757:errorcluster)  [unwired: 1 in]
        n189 = Close File(refnum=w756, error in=w757) -> (error out=w741:errorcluster)  [unwired: 1 out]
      }
      frame "output" {
        n190 = local read "Transfer/Output - Drain"() -> (w765:u32)
        n191 = local read "Transfer/Output - Source/Common"() -> (w764:u32)
        n192 = local read "Transfer/Output - Gate"() -> (w766:u32)
        n193 = Delete From Array(array=w864, index=0 ("Index")) -> (deleted portion=w862:string, array with subset deleted=w861:string[])  [unwired: 1 in]
        n194 = Bundle By Name(cluster=w777, "Emergency Stop"=w873) -> (w827:T1)
        n195 = Number To Decimal String(number=w823) -> (decimal integer string=w822:string)  [unwired: 1 in]
        n196 = case shown="\"d\", Default" w862 {
          tunnel: [w958 w959] -> w860
          frame "s" {
            w958 = u16 0 items=["Single", "Double"] ("sweep mode")
          }
          frame "d", Default {
            w959 = u16 1 items=["Single", "Double"] ("sweep mode")
          }
        }
        n197 = Fract/Exp String To Number(string=w861) -> (number=w846:dbl[])  [unwired: 3 in, 1 out]
        n198 = Concatenate Strings(w871, "-output-" ("Substring"), w822, w820, ".txt" ("Suffix (transfer)")) -> (w872:string)
        n199 = VISA Write(VISA resource name=w842, write buffer=":PAGE:CHAN:MODE SWE;" ("write buffer (\"\")"), error in (no error)=w841) -> (VISA resource name out=w839:refnum<visa-resource-name>, error out=w840:errorcluster)  [unwired: 1 out]
        n200 = String To Path(string=w872) -> (path=w870:path)
        n201 = Index Array(array=w846, index #1=0 ("Index")) -> (element #1=w859:dbl, element #2=w858:dbl, element #3=w857:dbl)  [unwired: 2 in]
        n202 = Delete From Array(array=w846, length=3 ("Length"), index=0 ("Index")) -> (array with subset deleted=w844:dbl[])  [unwired: 1 out]
        n203 = local read "Plot output curve extrema vs time"() -> (w774:bool)
        n204 = local read "Transfer/Output - Probe 4"() -> (w767:u32)
        n205 = Bundle By Name(cluster=w851, "Gate Start"=w859, "Gate Stop"=w858, "Gate Step (linear only)"=w857, "Gate Compliance"=w868, "Range mode"=w835, "Range"=w834) -> (w836:T6)
        n206 = case shown="True" w774 {
          tunnel: w819 -> [w875 w878]
          tunnel: w816 -> [_ w877]
          tunnel: [w875 w876] -> w793
          frame False {
          }
          frame True {
            n207 = Build Array (concatenate)(w878, w877) -> (w876:i32[])
          }
        }
        n208 = Index Array(array=w844, index #1=0 ("Index")) -> (element #1=w854:dbl, element #2=w853:dbl, element #3=w852:dbl)  [unwired: 2 in]
        n209 = call <vilib>:"compatOverwrite.vi"("overwrite (F)"=TRUE) -> ("overwrite?"=w826:T8)
        n210 = Bundle By Name(cluster=w850, "Drain Start"=w854, "Drain Stop"=w853, "Drain Step"=w852, "Drain Compliance"=w869, "Range mode"=w833, "Range"=w832) -> (w837:T7)
        n211 = call "4155C Output v3.0.vi"("VISA resource name in"=w839, "Source/Common"=w764, 2:"Gate"=w836, 3:"Drain"=w837, 4:"Drain"=w765, "Timings"=w867, "error in (no error)"=w840, 7:"Probe 4"=w773, 8:"Gate"=w766, 9:"Probe 4"=w767, "sweep mode"=w860, "Panel controls"=w827, "Standby"=w768) -> ("VD"=w825:dbl[], "Outparams"=w831:T9, "VISA Resource Name out"=w866:refnum<visa-resource-name>, "IS"=w803:dbl[], "ID"=w804:dbl[], "IG"=w802:dbl[], "error out"=w817:errorcluster, "Probe 4"=w828:dbl[])  [unwired: 7 in]
        n212 = Unbundle By Name(w831) -> ("V2 Step"=w830:dbl, "V2 Start"=w829:dbl, "Number of points"=w791:i32)
        n213 = call "4155C Split array.vi"("Number of VAR2 steps"=w791, "Y2 data in"=w804, "X data in"=w825, "Y1 data in"=w803, "Y3 data in"=w802, "error in (no error)"=w817) -> ("Array of clusters"=w818:cluster{"Y data in":dbl[], "X data in":dbl[]}[], "error out"=w779:errorcluster)  [unwired: 1 in]
        n214 = case shown="True" "Plot output curve extrema vs time" {
          tunnel: w824 -> [w887 w957]
          tunnel: w815 -> [w888 w952]
          tunnel: w806 -> [w882 w948]
          tunnel: w805 -> [w881 w947]
          tunnel: w804 -> [_ w944]
          tunnel: w803 -> [_ w942]
          tunnel: w802 -> [_ w941]
          tunnel: w801 -> [w889 w937]
          tunnel: w800 -> [w890 w936]
          tunnel: w799 -> [w885 w933]
          tunnel: w798 -> [w886 w932]
          tunnel: w797 -> [w883 w929]
          tunnel: w796 -> [w884 w928]
          tunnel: w795 -> [w879 w925]
          tunnel: w794 -> [w880 w924]
          tunnel: w793 -> [_ w917]
          tunnel: [w885 w912] -> w792
          tunnel: w791 -> [_ w911]
          tunnel: [w886 w910] -> w790
          tunnel: [w887 w909] -> w789
          tunnel: [w888 w908] -> w788
          tunnel: [w889 w907] -> w787
          tunnel: [w890 w906] -> w786
          tunnel: [w879 w905] -> w785
          tunnel: [w880 w904] -> w784
          tunnel: [w881 w903] -> w783
          tunnel: [w882 w902] -> w782
          tunnel: [w883 w901] -> w781
          tunnel: [w884 w900] -> w780
          tunnel: w779 -> [w891 w899]
          tunnel: [w891 w895] -> w778
          frame False {
          }
          frame True {
            # "Adjusts graph colors."
            # "Adjusts graph colors."
            # "Ion will be the middle element of the array. The calculation of the index is done only once, since Is, Id, and Ig have the same dimensions."
            # "abs(Ig)"
            # "abs(Is)"
            # "Y1: Is\nY2: Id\nY3: Ig"
            # "abs(Id)"
            # "Adjusts graph colors."
            # "Adjusts graph colors."
            # "Adjusts graph colors."
            n215 = Absolute Value(x=w942) -> (abs(x)=w927:dbl[])
            n216 = Absolute Value(x=w944) -> (abs(x)=w943:dbl[])
            n217 = Absolute Value(x=w941) -> (abs(x)=w930:dbl[])
            n218 = Array Size(array=w943) -> (size(s)=w951:i32)
            n219 = Divide(x=w951, y=2) -> (x/y=w894:dbl)
            n220 = Subtract(x=w894, y=1) -> (x-y=w893:dbl)
            n221 = Array Max & Min(array=w927) -> (max value=w934:dbl, min value=w935:dbl)  [unwired: 2 out]
            n222 = Array Max & Min(array=w943) -> (max value=w956:dbl, min value=w940:dbl)  [unwired: 2 out]
            n223 = Array Max & Min(array=w930) -> (max value=w939:dbl, min value=w938:dbl)  [unwired: 2 out]
            n224 = Index Array(array=w927, index=w893) -> (element=w918:dbl)
            n225 = Index Array(array=w927, index=0) -> (element=w919:dbl)
            n226 = Index Array(array=w943, index=w893) -> (element=w920:dbl)
            n227 = Index Array(array=w943, index=0) -> (element=w921:dbl)
            n228 = Index Array(array=w930, index=w893) -> (element=w923:dbl)
            n229 = Index Array(array=w930, index=0) -> (element=w922:dbl)
            n230 = local write "Ig max"(w939) -> ()
            n231 = local write "Ig min"(w938) -> ()
            n232 = local write "Is max"(w934) -> ()
            n233 = local write "Is min"(w935) -> ()
            n234 = local write "Id max"(w956) -> ()
            n235 = local write "Id min"(w940) -> ()
            n236 = Build Array (concatenate)(w933, w934) -> (w912:dbl[])
            n237 = Build Array (concatenate)(w932, w935) -> (w910:dbl[])
            n238 = local write "Is off"(w919) -> ()
            n239 = local write "Is on"(w918) -> ()
            n240 = Build Array (concatenate)(w957, w956) -> (w909:dbl[])
            n241 = Build Array (concatenate)(w952, w940) -> (w908:dbl[])
            n242 = Build Array (concatenate)(w937, w939) -> (w907:dbl[])
            n243 = Build Array (concatenate)(w936, w938) -> (w906:dbl[])
            n244 = Build Array (concatenate)(w925, w918) -> (w905:dbl[])
            n245 = Build Array (concatenate)(w924, w919) -> (w904:dbl[])
            n246 = Build Array (concatenate)(w947, w920) -> (w903:dbl[])
            n247 = Build Array (concatenate)(w948, w921) -> (w902:dbl[])
            n248 = Build Array (concatenate)(w929, w923) -> (w901:dbl[])
            n249 = Build Array (concatenate)(w928, w922) -> (w900:dbl[])
            n250 = local write "Ig off"(w922) -> ()
            n251 = local write "Ig on"(w923) -> ()
            n252 = local write "Id off"(w921) -> ()
            n253 = local write "Id on"(w920) -> ()
            n254 = control-ref of="Imax vs time"() -> (w946:refnum<vi>)
            n255 = control-ref of="Imin vs time"() -> (w945:refnum<vi>)
            n256 = control-ref of="Ion vs time"() -> (w914:refnum<vi>)
            n257 = control-ref of="Ioff vs time"() -> (w913:refnum<vi>)
            n258 = control-ref of="I vs Vg"() -> (w955:refnum<vi>)
            n259 = call "4155C Split array.vi"("Number of VAR2 steps"=w911, "Y2 data in"=w903, "X data in"=w917, "Y1 data in"=w905, "Y3 data in"=w901, "error in (no error)"=w899) -> ("Array of clusters"=w915:cluster{"Y data in":dbl[], "X data in":dbl[]}[], "error out"=w898:errorcluster)  [unwired: 1 in]
            n260 = call "4155C Split array.vi"("Number of VAR2 steps"=w911, "Y2 data in"=w902, "X data in"=w917, "Y1 data in"=w904, "Y3 data in"=w900, "error in (no error)"=w898) -> ("Array of clusters"=w916:cluster{"Y data in":dbl[], "X data in":dbl[]}[], "error out"=w897:errorcluster)  [unwired: 1 in]
            n261 = call "4155C Split array.vi"("Number of VAR2 steps"=w911, "Y2 data in"=w909, "X data in"=w917, "Y1 data in"=w912, "Y3 data in"=w907, "error in (no error)"=w897) -> ("Array of clusters"=w954:cluster{"Y data in":dbl[], "X data in":dbl[]}[], "error out"=w896:errorcluster)  [unwired: 1 in]
            n262 = call "4155C Split array.vi"("Number of VAR2 steps"=w911, "Y2 data in"=w908, "X data in"=w917, "Y1 data in"=w910, "Y3 data in"=w906, "error in (no error)"=w896) -> ("Array of clusters"=w953:cluster{"Y data in":dbl[], "X data in":dbl[]}[], "error out"=w895:errorcluster)  [unwired: 1 in]
            n263 = call "4155C Config Chart Colours.vi"("Numeric"=w911, "XY Graph 2"=w946) -> ()  [unwired: 6 in]
            n264 = call "4155C Config Chart Colours.vi"("Numeric"=w911, "XY Graph 2"=w945) -> ()  [unwired: 6 in]
            n265 = call "4155C Config Chart Colours.vi"("Numeric"=w911, "XY Graph 2"=w914) -> ()  [unwired: 6 in]
            n266 = call "4155C Config Chart Colours.vi"("Numeric"=w911, "XY Graph 2"=w913) -> ()  [unwired: 6 in]
            n267 = call "4155C Config Chart Colours.vi"("Numeric"=w911, "XY Graph 2"=w955) -> ()  [unwired: 6 in]
            n268 = local write "Imax vs time"(w954) -> ()
            n269 = local write "Imin vs time"(w953) -> ()
            n270 = local write "Ion vs time"(w915) -> ()
            n271 = local write "Ioff vs time"(w916) -> ()
          }
        }
        n272 = local write "I vs Vd"(w818) -> ()
        n273 = Open/Create/Replace File(file path (use dialog)=w870, error in=w778, operation (0:open)=w826) -> (refnum out=w813:refnum<file>, error out=w811:errorcluster)  [unwired: 3 in, 1 out]
        n274 = call "4155C Make Big 2d array.vi"("1D Var1"=w825, "1d IS"=w803, "1d ID"=w804, "1d IG"=w802, "1d SMU4"=w828, "SMU4"=w773, "VAR2 START"=w829, "Number of VAR2 steps"=w791, "VAR2 STEP"=w830, "VAR1 Name"="Vd", "Decimal places in header"=i8 1, "VAR2 Name"="Vg") -> ("Header array"=w814:string[], "Data array"=w812:dbl[][])  [unwired: 14 in]
        n275 = call "4155C Write array to file.vi"("Byte Stream File Refnum"=w813, "Header"=w814, "Data Array"=w812, "error in (no error)"=w811) -> ("dup refnum"=w810:refnum<file>, "error out"=w809:errorcluster)  [unwired: 1 in]
        n276 = Close File(refnum=w810, error in=w809) -> (error out=w865:errorcluster)  [unwired: 1 out]
      }
      frame "output-fpp" {
        n277 = local read "FPP - Source"() -> (w962:u32)
        n278 = local read "FPP - Drain"() -> (w963:u32)
        n279 = local read "FPP - Gate"() -> (w964:u32)
        n280 = Number To Decimal String(number=w984) -> (decimal integer string=w1038:string)  [unwired: 1 in]
        n281 = Bundle By Name(cluster=w1014, "Emergency Stop"=w1041) -> (w1051:T1)
        n282 = Delete From Array(array=w1029, index=0 ("Index")) -> (deleted portion=w1027:string, array with subset deleted=w1026:string[])  [unwired: 1 in]
        n283 = VISA Write(VISA resource name=w1005, write buffer=":PAGE:CHAN:MODE SWE;" ("write buffer (\"\")"), error in (no error)=w1002) -> (VISA resource name out=w1004:refnum<visa-resource-name>, error out=w1003:errorcluster)  [unwired: 1 out]
        n284 = Concatenate Strings(w1037, "-outputfpp-" ("Substring"), w1038, w983, ".txt" ("Substring")) -> (w1040:string)
        n285 = case shown="\"d\", Default" w1027 {
          tunnel: [w1052 w1053] -> w1025
          frame "s" {
            w1052 = u16 0 items=["Single", "Double"] ("sweep mode")
          }
          frame "d", Default {
            w1053 = u16 1 items=["Single", "Double"] ("sweep mode")
          }
        }
        n286 = Fract/Exp String To Number(string=w1026) -> (number=w1008:dbl[])  [unwired: 3 in, 1 out]
        n287 = String To Path(string=w1040) -> (path=w1036:path)
        n288 = Index Array(array=w1008, index #1=0 ("Index")) -> (element #1=w1024:dbl, element #2=w1023:dbl, element #3=w1022:dbl)  [unwired: 2 in]
        n289 = Delete From Array(array=w1008, length=3 ("Length"), index=0 ("Index")) -> (array with subset deleted=w1007:dbl[])  [unwired: 1 out]
        n290 = local read "FPP - Probe 1"() -> (w960:u32)
        n291 = local read "FPP - Probe 2"() -> (w961:u32)
        n292 = Bundle By Name(cluster=w1016, "Gate Start"=w1024, "Gate Stop"=w1023, "Gate Step (linear only)"=w1022, "Gate Compliance"=w1034, "Range mode"=w1000, "Range"=w999) -> (w1050:T6)
        n293 = Index Array(array=w1007, index #1=0 ("Index")) -> (element #1=w1019:dbl, element #2=w1018:dbl, element #3=w1017:dbl)  [unwired: 2 in]
        n294 = call <vilib>:"compatOverwrite.vi"("overwrite (F)"=TRUE) -> ("overwrite?"=w988:T8)
        n295 = Bundle By Name(cluster=w1015, "Drain Start"=w1019, "Drain Stop"=w1018, "Drain Step"=w1017, "Drain Compliance"=w1035, "Range mode"=w998, "Range"=w1001) -> (w1049:T7)
        n296 = call "4155C Output-FPP v3.0.vi"("VISA resource name in"=w1004, "FPP - Source"=w962, "Gate"=w1050, "Drain"=w1049, "FPP - Drain"=w963, "Timings"=w1033, "error in (no error)"=w1003, "FPP - Gate"=w964, "FPP - Probe 1"=w960, "sweep mode"=w1025, "FPP - Probe 2"=w961, "Panel controls"=w1051) -> ("VD"=w993:dbl[], "Outparams"=w996:T9, "VISA Resource Name out"=w1031:refnum<visa-resource-name>, "Vprobe2"=w992:dbl[], "ID"=w991:dbl[], "IG"=w990:dbl[], "Vprobe1"=w989:dbl[], "error out"=w1032:errorcluster)  [unwired: 8 in]
        n297 = Unbundle By Name(w996) -> ("V2 Step"=w997:dbl, "V2 Start"=w995:dbl, "Number of points"=w994:i32)
        n298 = Open/Create/Replace File(file path (use dialog)=w1036, error in=w1032, operation (0:open)=w988) -> (refnum out=w1046:refnum<file>, error out=w1047:errorcluster)  [unwired: 3 in, 1 out]
        n299 = call "4155C Make Big 2d array FPP.vi"("1D Var1"=w993, "1d ID"=w991, "1d Vp2"=w992, "1d IG"=w990, "1d Vp1"=w989, "VAR2 START"=w995, "Number of VAR2 steps"=w994, "VAR2 STEP"=w997, "VAR1 Name"="Vd", "Decimal places in header"=i8 1, "VAR2 Name"="Vg") -> ("Header array"=w1042:string[], "Data array"=w1043:dbl[][])  [unwired: 15 in]
        n300 = call "4155C Write array to file.vi"("Byte Stream File Refnum"=w1046, "Header"=w1042, "Data Array"=w1043, "error in (no error)"=w1047) -> ("dup refnum"=w1044:refnum<file>, "error out"=w1045:errorcluster)  [unwired: 1 in]
        n301 = Close File(refnum=w1044, error in=w1045) -> (error out=w1030:errorcluster)  [unwired: 1 out]
      }
      frame "itime" {
        n302 = Delete From Array(array=w1061, index=1) -> (deleted portion=w1060:string)  [unwired: 1 in, 1 out]
        n303 = Delete From Array(array=w1061, index=0 ("Index")) -> (deleted portion=w1089:string)  [unwired: 1 in, 1 out]
        n304 = Fract/Exp String To Number(string=w1060) -> (number=w1059:dbl)  [unwired: 3 in, 1 out]
        n305 = case shown="\"l\"" w1089 {
          tunnel: w1088 -> [w1094 w1096 w1100]
          tunnel: [w1093 w1095 w1099] -> w1081
          tunnel: w1059 -> [w1091 _ w1098]
          frame "s" {
            w1092 = u32 0 items=["short  ", "medium  ", "long  "] ("integration time 2")
            n306 = Bundle By Name(cluster=w1094, "integration time"=w1092, "Short/Long integration time"=w1091) -> (w1093:T4)
          }
          frame "m", Default {
            w1097 = u32 1 items=["short  ", "medium  ", "long  "] ("integration time 2")
            n307 = Bundle By Name(cluster=w1096, "integration time"=w1097) -> (w1095:T4)
          }
          frame "l" {
            w1101 = u32 2 items=["short  ", "medium  ", "long  "] ("integration time 2")
            n308 = Bundle By Name(cluster=w1100, "integration time"=w1101, "Short/Long integration time"=w1098) -> (w1099:T4)
          }
        }
      }
      frame "pulsed" {
        n309 = Delete From Array(array=w1134, index=0 ("Index")) -> (deleted portion=w1135:string, array with subset deleted=w1122:string[])  [unwired: 1 in]
        n310 = case shown="\"on\", Default" w1135 {
          tunnel: w1133 -> [w1145 w1148]
          tunnel: [w1144 w1147] -> w1126
          tunnel: w1122 -> [w1142 _]
          frame "on", Default {
            w1143 = u16 1 items=["Continuous", "Pulsed"] ("sweep method")
            n311 = Fract/Exp String To Number(string=w1142) -> (number=w1140:dbl[])  [unwired: 3 in, 1 out]
            n312 = Index Array(array=w1140, index #1=0 ("Index")) -> (element #1=w1139:dbl, element #2=w1138:dbl, element #3=w1137:dbl)  [unwired: 2 in]
            n313 = Bundle By Name(cluster=w1145, "sweep method"=w1143, "Pulse period"=w1139, "Base voltage"=w1138, "Pulse width"=w1137) -> (w1144:T4)
          }
          frame "off" {
            w1146 = u16 0 items=["Continuous", "Pulsed"] ("sweep method")
            n314 = Bundle By Name(cluster=w1148, "sweep method"=w1146) -> (w1147:T4)
          }
        }
      }
      frame "gaterangemode" {
        n315 = Delete From Array(array=w1179, index=0 ("Index")) -> (deleted portion=w1180:string)  [unwired: 1 in, 1 out]
        n316 = case shown="\"f\"" w1180 {
          tunnel: [w1182 w1183 w1184] -> w1169
          frame "a", Default {
            w1182 = u16 0 items=["Auto", "Limited", "Fixed"] ("Gate Range\nmode 2")
          }
          frame "f" {
            w1183 = u16 2 items=["Auto", "Limited", "Fixed"] ("Gate Range\nmode 2")
          }
          frame "l" {
            w1184 = u16 1 items=["Auto", "Limited", "Fixed"] ("Gate Range\nmode 2")
          }
        }
      }
      frame "gaterange" {
        (unwired) u8 11 items=["10fA  ", "100fA  ", "1nA  ", "10nA", "100nA", "1uA", "10uA", "100uA", "1mA", "10mA", "100mA", "1A"] ("Gate Range 2")
        n317 = Delete From Array(array=w1222, index=0 ("Index")) -> (deleted portion=w1212:string)  [unwired: 1 in, 1 out]
        n318 = Scan Value(string=w1212, format string="") -> (value=w1210:dbl)  [unwired: 1 in, 1 out]
        n319 = Logarithm Base 10(1:w1210) -> (0:w1209:dbl)
        n320 = Round To Nearest(number=w1209) -> (nearest integer value=w1208:dbl)
        n321 = Add(x=w1208, y=11.0) -> (x+y=w1206:dbl)
        n322 = To Unsigned Byte Integer(number=w1206) -> (unsigned 8bit integer=w1205:u8)
      }
      frame "drainrange" {
        (unwired) u8 11 items=["10fA  ", "100fA  ", "1nA  ", "10nA", "100nA", "1uA", "10uA", "100uA", "1mA", "10mA", "100mA", "1A"] ("Gate Range 2")
        n323 = Delete From Array(array=w1261, index=0 ("Index")) -> (deleted portion=w1252:string)  [unwired: 1 in, 1 out]
        n324 = Scan Value(string=w1252, format string="") -> (value=w1250:dbl)  [unwired: 1 in, 1 out]
        n325 = Logarithm Base 10(1:w1250) -> (0:w1249:dbl)
        n326 = Round To Nearest(number=w1249) -> (nearest integer value=w1248:dbl)
        n327 = Add(x=w1248, y=11.0) -> (x+y=w1246:dbl)
        n328 = To Unsigned Byte Integer(number=w1246) -> (unsigned 8bit integer=w1245:u8)
      }
      frame "drainrangemode" {
        n329 = Delete From Array(array=w1293, index=0 ("Index")) -> (deleted portion=w1294:string)  [unwired: 1 in, 1 out]
        n330 = case shown="\"f\"" w1294 {
          tunnel: [w1296 w1297 w1298] -> w1283
          frame "a", Default {
            w1296 = u16 0 items=["Auto", "Limited", "Fixed"] ("Gate Range\nmode 2")
          }
          frame "f" {
            w1297 = u16 2 items=["Auto", "Limited", "Fixed"] ("Gate Range\nmode 2")
          }
          frame "l" {
            w1298 = u16 1 items=["Auto", "Limited", "Fixed"] ("Gate Range\nmode 2")
          }
        }
      }
      frame "Error", Default {
      }
      frame "logfile" {
        n331 = Number To Decimal String(number=w1349) -> (decimal integer string=w1384:string)  [unwired: 1 in]
        n332 = Concatenate Strings(w1383, "logfile" ("Substring"), w1384, w1347, ".txt" ("Substring")) -> (w1381:string)
        n333 = String To Path(string=w1381) -> (path=w1354:path)
        n334 = Unbundle(w1380) -> ("integration time"=w1379:u32, "Short/Long integration time"=w1378:dbl, "hold time (sec)"=w1377:dbl, "delay time (sec)"=w1376:dbl, "Step Time (0 disables)"=w1375:dbl, "sweep method"=w1374:u16, "Pulse period"=w1373:dbl, "Base voltage"=w1372:dbl, "Pulse width"=w1371:dbl)
        n335 = Build Array(w1379, w1378, w1377, w1376, w1375, w1374, w1373, w1372, w1371, w1365, w1366, w1367, w1368, w1369, w1370) -> (w1358:dbl[])
        n336 = Insert Into Array(array=dbl[][] [] ("Input Array"), new element=w1358) -> (w1357:dbl[][])  [unwired: 2 in]
        n337 = call <vilib>:"compatOverwrite.vi"("overwrite (F)"=TRUE) -> ("overwrite?"=w1352:T8)
        n338 = Open/Create/Replace File(file path (use dialog)=w1354, error in=w1356, operation (0:open)=w1352) -> (refnum out=w1362:refnum<file>, error out=w1361:errorcluster)  [unwired: 3 in, 1 out]
        n339 = call "4155C Write array to file.vi"("Byte Stream File Refnum"=w1362, "Header"=string[] ["Int Time", "Short/Long Itime", "Hold time", "Delay time", "Step time", "Sweep method", "Pulse period", "Base Voltage", "Pulse width", "Drain compliance", "Gate compliance", "Gate range mode", "Gate range", "S/D range mode", "S/D range"], "Data Array"=w1357, "error in (no error)"=w1361) -> ("dup refnum"=w1364:refnum<file>, "error out"=w1363:errorcluster)  [unwired: 1 in]
        n340 = Close File(refnum=w1364, error in=w1363) -> (error out=w1355:errorcluster)  [unwired: 1 out]
      }
      frame "sample" {
        w1408 = 1
        # "Add a time offset (elapsed time) to the time axis."
        # "Adjusts graph colors."
        n341 = Number To Decimal String(number=w1440) -> (decimal integer string=w1482:string)  [unwired: 1 in]
        n342 = Fract/Exp String To Number(string=w1479) -> (number=w1444:dbl[])  [unwired: 3 in, 1 out]
        n343 = local read "Sample - Probe 4"() -> (w1390:u32)
        n344 = Concatenate Strings(w1460, "-sample-" ("Substring"), w1482, w1438, ".txt" ("Substring")) -> (w1480:string)
        n345 = local read "Sample - Drain"() -> (w1391:u32)
        n346 = Index Array(array=w1444, index=0 ("Index")) -> (element=w1477:dbl)
        n347 = String To Path(string=w1480) -> (path=w1464:path)
        n348 = Index Array(array=w1444, index=2 ("Index")) -> (element=w1473:dbl)
        n349 = Index Array(array=w1444, index=3 ("Index")) -> (element=w1446:dbl)
        n350 = Index Array(array=w1444, index=4 ("Index")) -> (element=w1443:dbl)
        n351 = Index Array(array=w1444, index=1 ("Index")) -> (element=w1474:dbl)
        n352 = local read "Plot sample extrema vs time"() -> (w1411:bool)
        n353 = local read "Time Units"() -> (w1386:u16)
        n354 = local read "Sample - Gate"() -> (w1393:u32)
        n355 = local read "Sample - Source/Common"() -> (w1392:u32)
        n356 = call "4155C Config Sampling Measurements v3.0.vi"("VISA session"=w1485, "Num Points"=w1473, "Sample - Drain"=w1391, "Display on/off"=TRUE, "Gate Compliance"=w1461, "Sampling interval"=w1443, "Sample - Source/Common"=w1392, "Sample - Probe 4"=w1390, "Drain Compliance"=w1483, "Standby"=w1394, "error in (no error)"=w1484, "Timings"=w1452, "Sample - Gate"=w1393, "Sample time"=w1446) -> ("dup VISA resource name"=w1487:refnum<visa-resource-name>, "error out"=w1486:errorcluster)
        n357 = call "4155C Take Sample v3.0.vi"("VISA resource name in"=w1487, "Emergency Stop"=w1457, "Sample - Gate"=w1393, "Vg"=w1477, "Sample - Drain"=w1391, "Vd"=w1474, "error in (no error)"=w1486) -> ("Time"=w1388:dbl[], "VISA Resource Name out"=w1454:refnum<visa-resource-name>, "Ig"=w1404:dbl[], "Id"=w1405:dbl[], "Is"=w1406:dbl[], "error out"=w1409:errorcluster)  [unwired: 3 in]
        n358 = case shown="0, Default" w1386 {
          tunnel: [w1490 w1491 w1494] -> w1389
          tunnel: w1388 -> [w1489 w1491 w1493]
          frame 2 {
            n359 = Divide(x=w1489, y=3600.0) -> (x/y=w1490:dbl[])
          }
          frame 0, Default {
          }
          frame 1 {
            n360 = Divide(x=w1493, y=60.0) -> (x/y=w1494:dbl[])
          }
        }
        n361 = Insert Into Array(array=w1402, new element=w1405) -> (w1396:dbl[])  [unwired: 1 in]
        n362 = Add(x=w1389, y=w1387) -> (x+y=w1407:dbl[])
        n363 = Insert Into Array(array=w1401, new element=w1406) -> (w1397:dbl[])  [unwired: 1 in]
        n364 = Insert Into Array(array=w1403, new element=w1404) -> (w1399:dbl[])  [unwired: 1 in]
        n365 = case shown="True" w1411 {
          tunnel: w1412 -> [w1495 w1497]
          tunnel: [w1495 w1498] -> w1410
          tunnel: w1407 -> [_ w1496]
          frame False {
          }
          frame True {
            n366 = Insert Into Array(array=w1497, new element=w1496) -> (w1498:i32[])  [unwired: 1 in]
          }
        }
        n367 = case shown="True" "Plot sample extrema vs time" {
          tunnel: w1406 -> [_ w1526]
          tunnel: w1405 -> [_ w1527]
          tunnel: w1404 -> [_ w1528]
          tunnel: [w1505 w1515] -> w1395
          tunnel: w1409 -> [w1505 w1519]
          tunnel: w1433 -> [w1504 w1531]
          tunnel: w1432 -> [w1503 w1530]
          tunnel: w1431 -> [w1502 w1532]
          tunnel: w1430 -> [w1501 w1529]
          tunnel: w1429 -> [w1500 w1534]
          tunnel: w1428 -> [w1499 w1533]
          tunnel: [w1504 w1517] -> w1427
          tunnel: [w1503 w1510] -> w1426
          tunnel: [w1502 w1511] -> w1425
          tunnel: [w1501 w1535] -> w1424
          tunnel: [w1500 w1518] -> w1423
          tunnel: [w1499 w1512] -> w1422
          tunnel: w1410 -> [_ w1506]
          frame False {
          }
          frame True {
            w1513 = 1
            # "Number of VAR2 steps is 1."
            # "abs(Ig)"
            # "abs(Is)"
            # "abs(Id)"
            # "Adjusts graph colors."
            n368 = Absolute Value(x=w1528) -> (abs(x)=w1507:dbl[])
            n369 = Absolute Value(x=w1527) -> (abs(x)=w1508:dbl[])
            n370 = Absolute Value(x=w1526) -> (abs(x)=w1509:dbl[])
            n371 = Array Max & Min(array=w1509) -> (max value=w1525:dbl, min value=w1522:dbl)  [unwired: 2 out]
            n372 = Array Max & Min(array=w1508) -> (max value=w1524:dbl, min value=w1521:dbl)  [unwired: 2 out]
            n373 = Array Max & Min(array=w1507) -> (max value=w1523:dbl, min value=w1520:dbl)  [unwired: 2 out]
            n374 = local write "Id max"(w1524) -> ()
            n375 = local write "Id min"(w1521) -> ()
            n376 = local write "Ig max"(w1523) -> ()
            n377 = local write "Ig min"(w1520) -> ()
            n378 = Insert Into Array(array=w1534, new element=w1507) -> (w1518:dbl[])  [unwired: 1 in]
            n379 = Insert Into Array(array=w1533, new element=w1507) -> (w1512:dbl[])  [unwired: 1 in]
            n380 = local write "Is max"(w1525) -> ()
            n381 = local write "Is min"(w1522) -> ()
            n382 = Insert Into Array(array=w1532, new element=w1508) -> (w1511:dbl[])  [unwired: 1 in]
            n383 = Insert Into Array(array=w1529, new element=w1508) -> (w1535:dbl[])  [unwired: 1 in]
            n384 = Insert Into Array(array=w1531, new element=w1509) -> (w1517:dbl[])  [unwired: 1 in]
            n385 = Insert Into Array(array=w1530, new element=w1509) -> (w1510:dbl[])  [unwired: 1 in]
            n386 = control-ref of="Imax vs time"() -> (w1536:refnum<vi>)
            n387 = call "4155C Config Chart Colours.vi"("Numeric"=w1513, "XY Graph 2"=w1536) -> ()  [unwired: 6 in]
            n388 = call "4155C Split array.vi"("Number of VAR2 steps"=w1513, "Y2 data in"=w1511, "X data in"=w1506, "Y1 data in"=w1517, "Y3 data in"=w1518, "error in (no error)"=w1519) -> ("Array of clusters"=w1537:cluster{"Y data in":dbl[], "X data in":dbl[]}[], "error out"=w1516:errorcluster)  [unwired: 1 in]
            n389 = call "4155C Split array.vi"("Number of VAR2 steps"=w1513, "Y2 data in"=w1511, "X data in"=w1506, "Y1 data in"=w1510, "Y3 data in"=w1512, "error in (no error)"=w1516) -> ("Array of clusters"=w1514:cluster{"Y data in":dbl[], "X data in":dbl[]}[], "error out"=w1515:errorcluster)  [unwired: 1 in]
            n390 = local write "Imax vs time"(w1537) -> ()
            n391 = local write "Imin vs time"(w1514) -> ()
          }
        }
        n392 = Insert Into Array(array=w1400, new element=w1407) -> (w1398:dbl[])  [unwired: 1 in]
        n393 = control-ref of="I vs time (Bias Stress)"() -> (w1415:refnum<vi>)
        n394 = call "4155C Split array.vi"("Number of VAR2 steps"=w1408, "Y2 data in"=w1396, "X data in"=w1398, "Y1 data in"=w1397, "Y3 data in"=w1399) -> ("Array of clusters"=w1414:cluster{"Y data in":dbl[], "X data in":dbl[]}[])  [unwired: 2 in, 1 out]
        n395 = call "4155C Config Chart Colours.vi"("Numeric"=w1408, "XY Graph 2"=w1415) -> ()  [unwired: 6 in]
        n396 = local write "I vs time (Bias Stress)"(w1414) -> ()
        n397 = Insert Into Array(array=dbl[][] [] ("Input Array"), new element=w1407) -> (w1413:dbl[][])  [unwired: 2 in]
        n398 = Insert Into Array(array=w1413, new element=w1404) -> (w1467:dbl[][])  [unwired: 2 in]
        n399 = VISA Write(VISA resource name=w1454, write buffer=":DISP ON" ("write buffer (\"\")"), error in (no error)=w1395) -> (VISA resource name out=w1453:refnum<visa-resource-name>, error out=w1455:errorcluster)  [unwired: 1 out]
        n400 = Insert Into Array(array=w1467, new element=w1405) -> (w1466:dbl[][])  [unwired: 2 in]
        n401 = Insert Into Array(array=w1466, new element=w1406) -> (w1459:dbl[][])  [unwired: 2 in]
        n402 = Transpose 2D Array(2D array=w1459) -> (transposed array=w1458:dbl[][])
        n403 = call <vilib>:"compatOverwrite.vi"("overwrite (F)"=TRUE) -> ("overwrite?"=w1441:T8)
        n404 = Open/Create/Replace File(file path (use dialog)=w1464, error in=w1455, operation (0:open)=w1441) -> (refnum out=w1470:refnum<file>, error out=w1469:errorcluster)  [unwired: 3 in, 1 out]
        n405 = call "4155C Write array to file.vi"("Byte Stream File Refnum"=w1470, "Header"=string[] ["Time /Units", "Ig /A", "Id /A", "Is /A"], "Data Array"=w1458, "error in (no error)"=w1469) -> ("dup refnum"=w1472:refnum<file>, "error out"=w1471:errorcluster)  [unwired: 1 in]
        n406 = Close File(refnum=w1472, error in=w1471) -> (error out=w1462:errorcluster)  [unwired: 1 out]
      }
      frame "samplei" {
        n407 = local read "Sample I - Source/Common"() -> (w1538:u32)
        n408 = Number To Decimal String(number=w1563) -> (decimal integer string=w1614:string)  [unwired: 1 in]
        n409 = local read "Sample I - Probe 4 (Disabled)"() -> (w1541:u32)
        n410 = Concatenate Strings(w1593, "-samplei-" ("Substring"), w1614, w1562, ".txt" ("Substring")) -> (w1612:string)
        n411 = Fract/Exp String To Number(string=w1611) -> (number=w1578:dbl[])  [unwired: 3 in, 1 out]
        n412 = String To Path(string=w1612) -> (path=w1596:path)
        n413 = local read "Sample I - Probe 3 (Disabled)"() -> (w1540:u32)
        n414 = Index Array(array=w1578, index=4 ("Index")) -> (element=w1572:dbl)
        n415 = Index Array(array=w1578, index=3 ("Index")) -> (element=w1573:dbl)
        n416 = Index Array(array=w1578, index=1 ("Index")) -> (element=w1575:dbl)
        n417 = Index Array(array=w1578, index=0 ("Index")) -> (element=w1576:dbl)
        n418 = Index Array(array=w1578, index=2 ("Index")) -> (element=w1574:dbl)
        n419 = local read "Sample I - Drain/Gate"() -> (w1539:u32)
        n420 = call "4155C Config SamplingI Measurements v3.0.vi"("VISA session"=w1617, "Num Points"=w1575, "Sample I - Probe 3 (Disabled)"=w1540, "Display on/off"=TRUE, "Sample I - Source/Common"=w1538, "Sample I - Drain/Gate"=w1539, "Sampling interval"=w1573, "Standby"=w1542, "error in (no error)"=w1616, "Timings"=w1585, "Sample I - Probe 4 (Disabled)"=w1541, "Sample time"=w1574) -> ("dup VISA resource name"=w1619:refnum<visa-resource-name>, "error out"=w1618:errorcluster)  [unwired: 2 in]
        n421 = call "4155C Take SampleI v3.0.vi"("Sample I - Drain/Gate"=w1539, "Emergency Stop"=w1590, "error in (no error)"=w1618, "Idg 2"=w1576, "Vdg compliance 2"=w1572, "VISA resource name in"=w1619) -> ("error out"=w1588:errorcluster, "Idg"=w1621:dbl[], "Vdg"=w1598:dbl[], "VISA Resource Name out"=w1586:refnum<visa-resource-name>, "Is"=w1620:dbl[], "Time"=w1602:dbl[])
        n422 = Insert Into Array(array=dbl[][] [] ("Input Array"), new element=w1602) -> (w1601:dbl[][])  [unwired: 2 in]
        n423 = Insert Into Array(array=w1601, new element=w1598) -> (w1600:dbl[][])  [unwired: 2 in]
        n424 = Insert Into Array(array=w1600, new element=w1621) -> (w1599:dbl[][])  [unwired: 2 in]
        n425 = VISA Write(VISA resource name=w1586, write buffer=":DISP ON" ("write buffer (\"\")"), error in (no error)=w1588) -> (VISA resource name out=w1571:refnum<visa-resource-name>, error out=w1587:errorcluster)  [unwired: 1 out]
        n426 = Insert Into Array(array=w1599, new element=w1620) -> (w1592:dbl[][])  [unwired: 2 in]
        n427 = call <vilib>:"compatOverwrite.vi"("overwrite (F)"=TRUE) -> ("overwrite?"=w1566:T8)
        n428 = Open/Create/Replace File(file path (use dialog)=w1596, error in=w1587, operation (0:open)=w1566) -> (refnum out=w1605:refnum<file>, error out=w1604:errorcluster)  [unwired: 3 in, 1 out]
        n429 = Transpose 2D Array(2D array=w1592) -> (transposed array=w1591:dbl[][])
        n430 = call "4155C Write array to file.vi"("Byte Stream File Refnum"=w1605, "Header"=string[] ["Time /s", "Vdg /V", "Idg /A", "Is /A"], "Data Array"=w1591, "error in (no error)"=w1604) -> ("dup refnum"=w1607:refnum<file>, "error out"=w1606:errorcluster)  [unwired: 1 in]
        n431 = Close File(refnum=w1607, error in=w1606) -> (error out=w1569:errorcluster)  [unwired: 1 out]
        n432 = VISA Write(VISA resource name=w1571, write buffer=";:PAGE:SCON:STAN OFF;:PAGE:CHAN:VSU2:DIS;" ("write buffer (\"\")"), error in (no error)=w1569) -> (VISA resource name out=w1567:refnum<visa-resource-name>, error out=w1568:errorcluster)  [unwired: 1 out]
      }
      frame "#" {
        n433 = VISA Write(VISA resource name=w1646, write buffer=":DISP ON" ("write buffer (\"\")"), error in (no error)=w1645) -> (VISA resource name out=w1644:refnum<visa-resource-name>, error out=w1643:errorcluster)  [unwired: 1 out]
      }
      frame "stressV" {
        n434 = Number To Decimal String(number=w1677) -> (decimal integer string=w1718:string)  [unwired: 1 in]
        n435 = Concatenate Strings(w1702, "-stressV-" ("Substring"), w1718, w1676, ".txt" ("Substring")) -> (w1716:string)
        n436 = Fract/Exp String To Number(string=w1715) -> (number=w1688:dbl[])  [unwired: 3 in, 1 out]
        n437 = local read "Stress V - Drain"() -> (w1655:u32)
        n438 = String To Path(string=w1716) -> (path=w1706:path)
        n439 = Index Array(array=w1688, index=3 ("Index")) -> (element=w1685:dbl)
        n440 = Index Array(array=w1688, index=1 ("Index")) -> (element=w1683:dbl)
        n441 = Index Array(array=w1688, index=0 ("Index")) -> (element=w1682:dbl)
        n442 = Index Array(array=w1688, index=4 ("Index")) -> (element=w1687:dbl)
        n443 = Index Array(array=w1688, index=2 ("Index")) -> (element=w1684:dbl)
        n444 = local read "Stress V - Gate"() -> (w1656:u32)
        n445 = local read "Stress V - Source/Common"() -> (w1657:u32)
        n446 = call "4155C Config V Stress v3.0.vi"("Display on/off"=TRUE, "Stress V - Gate"=w1656, "Stress V - Drain"=w1655, "Stress V - Source/Common"=w1657, "IG compliance"=w1684, "ID compliance"=w1685, "error in (no error)"=w1720, "VG"=w1682, "VD"=w1683, "VISA session"=w1721) -> ("error out"=w1722:errorcluster, "dup VISA resource name"=w1723:refnum<visa-resource-name>)
        n447 = call "4155C Apply Stress.vi"("error in (no error)"=w1722, "Duration"=w1687, "Emergency Stop"=w1701, "VISA resource name in"=w1723) -> ("error out"=w1699:errorcluster, "VISA Resource Name out"=w1697:refnum<visa-resource-name>)
        n448 = VISA Write(VISA resource name=w1697, write buffer=":DISP ON" ("write buffer (\"\")"), error in (no error)=w1699) -> (VISA resource name out=w1696:refnum<visa-resource-name>, error out=w1698:errorcluster)  [unwired: 1 out]
        n449 = call <vilib>:"compatOverwrite.vi"("overwrite (F)"=TRUE) -> ("overwrite?"=w1681:T8)
        n450 = Open/Create/Replace File(file path (use dialog)=w1706, error in=w1698, operation (0:open)=w1681) -> (refnum out=w1709:refnum<file>, error out=w1708:errorcluster)  [unwired: 3 in, 1 out]
        n451 = call "4155C Write array to file.vi"("Byte Stream File Refnum"=w1709, "Header"=string[] ["V stress completed successfully", ""], "error in (no error)"=w1708) -> ("dup refnum"=w1711:refnum<file>, "error out"=w1710:errorcluster)  [unwired: 2 in]
        n452 = Close File(refnum=w1711, error in=w1710) -> (error out=w1704:errorcluster)  [unwired: 1 out]
      }
      frame "stressI" {
        n453 = Number To Decimal String(number=w1745) -> (decimal integer string=w1782:string)  [unwired: 1 in]
        n454 = Concatenate Strings(w1766, "-stressI-" ("Substring"), w1782, w1744, ".txt" ("Substring")) -> (w1780:string)
        n455 = Fract/Exp String To Number(string=w1779) -> (number=w1754:dbl[])  [unwired: 3 in, 1 out]
        n456 = local read "Stress I - Source/Common"() -> (w1724:u32)
        n457 = Index Array(array=w1754, index=1 ("Index")) -> (element=w1750:dbl)
        n458 = Index Array(array=w1754, index=0 ("Index")) -> (element=w1751:dbl)
        n459 = Index Array(array=w1754, index=2 ("Index")) -> (element=w1752:dbl)
        n460 = String To Path(string=w1780) -> (path=w1770:path)
        n461 = local read "Stress I - Drain/Gate"() -> (w1725:u32)
        n462 = call "4155C Config I Stress v3.0.vi"("Stress I - Drain/Gate"=w1725, "Stress I - Source/Common"=w1724, "Display on/off"=TRUE, "error in (no error)"=w1784, "VDG compliance"=w1750, "IDG"=w1751, "VISA session"=w1785) -> ("error out"=w1786:errorcluster, "dup VISA resource name"=w1787:refnum<visa-resource-name>)  [unwired: 1 in]
        n463 = call "4155C Apply Stress.vi"("error in (no error)"=w1786, "Duration"=w1752, "Emergency Stop"=w1765, "VISA resource name in"=w1787) -> ("error out"=w1763:errorcluster, "VISA Resource Name out"=w1761:refnum<visa-resource-name>)
        n464 = VISA Write(VISA resource name=w1761, write buffer=":DISP ON" ("write buffer (\"\")"), error in (no error)=w1763) -> (VISA resource name out=w1760:refnum<visa-resource-name>, error out=w1762:errorcluster)  [unwired: 1 out]
        n465 = call <vilib>:"compatOverwrite.vi"("overwrite (F)"=TRUE) -> ("overwrite?"=w1749:T8)
        n466 = Open/Create/Replace File(file path (use dialog)=w1770, error in=w1762, operation (0:open)=w1749) -> (refnum out=w1773:refnum<file>, error out=w1772:errorcluster)  [unwired: 3 in, 1 out]
        n467 = call "4155C Write array to file.vi"("Byte Stream File Refnum"=w1773, "Header"=string[] ["I stress completed successfully", ""], "error in (no error)"=w1772) -> ("dup refnum"=w1775:refnum<file>, "error out"=w1774:errorcluster)  [unwired: 2 in]
        n468 = Close File(refnum=w1775, error in=w1774) -> (error out=w1768:errorcluster)  [unwired: 1 out]
      }
      frame "vsu2pulse" {
        n469 = Number To Decimal String(number=w1808) -> (decimal integer string=w1843:string)  [unwired: 1 in]
        n470 = Concatenate Strings(w1828, "-vsu2-" ("Substring"), w1843, w1807, ".txt" ("Substring")) -> (w1841:string)
        n471 = Fract/Exp String To Number(string=w1840) -> (number=w1816:dbl[])  [unwired: 3 in, 1 out]
        n472 = String To Path(string=w1841) -> (path=w1832:path)
        n473 = Index Array(array=w1816, index=1 ("Index")) -> (element=w1815:dbl)
        n474 = Index Array(array=w1816, index=0 ("Index")) -> (element=w1813:dbl)
        n475 = local read "VSU2 Stress - Source/Common"() -> (w1788:u32)
        n476 = call "4155C Config VSU2 Stress v3.0.vi"("VISA session"=w1846, "Display on/off"=TRUE, "VSU2"=w1813, "error in (no error)"=w1845, "VSU2 Stress - Source/Common"=w1788) -> ("dup VISA resource name"=w1848:refnum<visa-resource-name>, "error out"=w1847:errorcluster)
        n477 = call "4155C Apply Stress.vi"("error in (no error)"=w1847, "Duration"=w1815, "Emergency Stop"=w1827, "VISA resource name in"=w1848) -> ("error out"=w1825:errorcluster, "VISA Resource Name out"=w1823:refnum<visa-resource-name>)
        n478 = VISA Write(VISA resource name=w1823, write buffer=":DISP ON" ("write buffer (\"\")"), error in (no error)=w1825) -> (VISA resource name out=w1822:refnum<visa-resource-name>, error out=w1824:errorcluster)  [unwired: 1 out]
        n479 = call <vilib>:"compatOverwrite.vi"("overwrite (F)"=TRUE) -> ("overwrite?"=w1812:T8)
        n480 = Open/Create/Replace File(file path (use dialog)=w1832, error in=w1824, operation (0:open)=w1812) -> (refnum out=w1835:refnum<file>, error out=w1834:errorcluster)  [unwired: 3 in, 1 out]
        n481 = call "4155C Write array to file.vi"("Byte Stream File Refnum"=w1835, "Header"=string[] ["VSU2 pulse completed successfully", ""], "error in (no error)"=w1834) -> ("dup refnum"=w1837:refnum<file>, "error out"=w1836:errorcluster)  [unwired: 2 in]
        n482 = Close File(refnum=w1837, error in=w1836) -> (error out=w1830:errorcluster)  [unwired: 1 out]
      }
      frame "sample-fpp" {
        w1884 = string[] ["Time /s", "Id VgVd /A", "Ig VgVd /A", "Vp1 VgVd /V", "Vp2 VgVd /V"] ("Header")
        w1888 = "%d" ("format string")
        n483 = local read "FPP - Drain"() -> (w1850:u32)
        n484 = local read "FPP - Source"() -> (w1849:u32)
        n485 = Fract/Exp String To Number(string=w1933) -> (number=w1921:dbl[])  [unwired: 3 in, 1 out]
        n486 = local read "FPP - Probe 1"() -> (w1853:u32)
        n487 = Number To Decimal String(number=w1874) -> (decimal integer string=w1936:string)  [unwired: 1 in]
        n488 = Concatenate Strings(w1927, "-samplefpp-" ("Substring"), w1936, w1873, ".txt" ("Substring")) -> (w1934:string)
        n489 = local read "FPP - Gate"() -> (w1851:u32)
        n490 = String To Path(string=w1934) -> (path=w1896:path)
        n491 = local read "FPP - Probe 2"() -> (w1852:u32)
        n492 = Index Array(array=w1921, index=0 ("Index")) -> (element=w1883:dbl)
        n493 = Index Array(array=w1921, index=1 ("Index")) -> (element=w1882:dbl)
        n494 = Index Array(array=w1921, index=2 ("Index")) -> (element=w1929:dbl)
        n495 = Index Array(array=w1921, index=3 ("Index")) -> (element=w1919:dbl)
        n496 = call "4155C Config Sampling Measurements FPP v3.0.vi"("VISA session"=w1939, "Gate Compliance"=w1928, "FPP - Source"=w1849, "FPP - Drain"=w1850, "Drain Compliance"=w1937, "error in (no error)"=w1938, "Num Points"=w1929, "Timings"=w1926, "FPP - Gate"=w1851, "FPP - Probe 1"=w1853, "Vg"=w1883, "Vd"=w1882, "Display on/off"=TRUE, "Sample time"=w1919, "FPP - Probe 2"=w1852, "Standby"=w1854) -> ("dup VISA resource name"=w1898:refnum<visa-resource-name>, "error out"=w1897:errorcluster)  [unwired: 2 in]
        n497 = Number To Decimal String(number=w1883) -> (decimal integer string=w1908:string)  [unwired: 1 in]
        n498 = call "4155C Take Sample FPP.vi"("VISA resource name in"=w1898, "error in (no error)"=w1897, "Emergency Stop"=w1899) -> ("Time"=w1903:dbl[], "Vp1"=w1913:dbl[], "VISA Resource Name out"=w1880:refnum<visa-resource-name>, "Ig"=w1901:dbl[], "Id"=w1902:dbl[], "Vp2"=w1911:dbl[], "error out"=w1900:errorcluster)  [unwired: 10 in]
        n499 = Insert Into Array(array=dbl[][] [] ("Input Array"), new element=w1903) -> (w1917:dbl[][])  [unwired: 2 in]
        n500 = Number To Decimal String(number=w1882) -> (decimal integer string=w1906:string)  [unwired: 1 in]
        n501 = Insert Into Array(array=w1917, new element=w1902) -> (w1916:dbl[][])  [unwired: 2 in]
        n502 = Concatenate Strings("(Vg = " ("Substring"), w1908, "V, Vd = " ("Substring"), w1906, "V)" ("Substring")) -> (w1904:string)
        n503 = Insert Into Array(array=w1916, new element=w1901) -> (w1915:dbl[][])  [unwired: 2 in]
        n504 = Insert Into Array(array=w1915, new element=w1913) -> (w1912:dbl[][])  [unwired: 2 in]
        n505 = Insert Into Array(array=w1912, new element=w1911) -> (w1881:dbl[][])  [unwired: 2 in]
        n506 = Transpose 2D Array(2D array=w1881) -> (transposed array=w1910:dbl[][])
        n507 = call <vilib>:"compatOverwrite.vi"("overwrite (F)"=TRUE) -> ("overwrite?"=w1878:T8)
        n508 = Open/Create/Replace File(file path (use dialog)=w1896, error in=w1900, operation (0:open)=w1878) -> (refnum out=w1893:refnum<file>, error out=w1894:errorcluster)  [unwired: 3 in, 1 out]
        n509 = Array To Spreadsheet String(array=w1884, 3:w1888) -> (spreadsheet string=w1890:string)  [unwired: 1 in]
        n510 = Search and Replace String(replace all?=TRUE ("replace all? (F)"), input string=w1890, search string="VgVd", replace string=w1904) -> (result string=w1886:string)  [unwired: 4 in, 3 out]
        n511 = Spreadsheet String To Array(format string=w1888, spreadsheet string=w1886, array type (2D Dbl)=w1884) -> (array=w1885:string[])  [unwired: 1 in]
        n512 = call "4155C Write array to file.vi"("Byte Stream File Refnum"=w1893, "Header"=w1885, "Data Array"=w1910, "error in (no error)"=w1894) -> ("dup refnum"=w1891:refnum<file>, "error out"=w1892:errorcluster)  [unwired: 1 in]
        n513 = Close File(refnum=w1891, error in=w1892) -> (error out=w1879:errorcluster)  [unwired: 1 out]
      }
      frame "resample-fpp" {
        w1972 = string[] ["Time /s", "Id VgVd /A", "Ig VgVd /A", "Vp1 VgVd /V", "Vp2 VgVd /V"] ("Header")
        w1976 = "%d" ("format string")
        n514 = Number To Decimal String(number=w1958) -> (decimal integer string=w2016:string)  [unwired: 1 in]
        n515 = Fract/Exp String To Number(string=w2013) -> (number=w1965:dbl[])  [unwired: 3 in, 1 out]
        n516 = Concatenate Strings(w2009, "-resamplefpp-" ("Substring"), w2016, w1959, ".txt" ("Substring")) -> (w2014:string)
        n517 = String To Path(string=w2014) -> (path=w1984:path)
        n518 = Index Array(array=w1965, index=0 ("Index")) -> (element=w1971:dbl)
        n519 = Index Array(array=w1965, index=1 ("Index")) -> (element=w1970:dbl)
        n520 = Number To Decimal String(number=w1971) -> (decimal integer string=w1994:string)  [unwired: 1 in]
        n521 = call "4155C Take Sample FPP.vi"("VISA resource name in"=w1967, "error in (no error)"=w1966, "Emergency Stop"=w1985) -> ("Time"=w1989:dbl[], "Vp1"=w1999:dbl[], "VISA Resource Name out"=w1969:refnum<visa-resource-name>, "Ig"=w1987:dbl[], "Id"=w1988:dbl[], "Vp2"=w1997:dbl[], "error out"=w1986:errorcluster)  [unwired: 10 in]
        n522 = Insert Into Array(array=dbl[][] [] ("Input Array"), new element=w1989) -> (w2003:dbl[][])  [unwired: 2 in]
        n523 = Number To Decimal String(number=w1970) -> (decimal integer string=w1992:string)  [unwired: 1 in]
        n524 = Insert Into Array(array=w2003, new element=w1988) -> (w2002:dbl[][])  [unwired: 2 in]
        n525 = Concatenate Strings("(Vg = " ("Substring"), w1994, "V, Vd = " ("Substring"), w1992, "V)" ("Substring")) -> (w1990:string)
        n526 = Insert Into Array(array=w2002, new element=w1987) -> (w2001:dbl[][])  [unwired: 2 in]
        n527 = Insert Into Array(array=w2001, new element=w1999) -> (w1998:dbl[][])  [unwired: 2 in]
        n528 = Insert Into Array(array=w1998, new element=w1997) -> (w1964:dbl[][])  [unwired: 2 in]
        n529 = call <vilib>:"compatOverwrite.vi"("overwrite (F)"=TRUE) -> ("overwrite?"=w1963:T8)
        n530 = Open/Create/Replace File(file path (use dialog)=w1984, error in=w1986, operation (0:open)=w1963) -> (refnum out=w1981:refnum<file>, error out=w1982:errorcluster)  [unwired: 3 in, 1 out]
        n531 = Array To Spreadsheet String(array=w1972, 3:w1976) -> (spreadsheet string=w1978:string)  [unwired: 1 in]
        n532 = Transpose 2D Array(2D array=w1964) -> (transposed array=w1996:dbl[][])
        n533 = Search and Replace String(replace all?=TRUE ("replace all? (F)"), input string=w1978, search string="VgVd", replace string=w1990) -> (result string=w1974:string)  [unwired: 4 in, 3 out]
        n534 = Spreadsheet String To Array(format string=w1976, spreadsheet string=w1974, array type (2D Dbl)=w1972) -> (array=w1973:string[])  [unwired: 1 in]
        n535 = call "4155C Write array to file.vi"("Byte Stream File Refnum"=w1981, "Header"=w1973, "Data Array"=w1996, "error in (no error)"=w1982) -> ("dup refnum"=w1979:refnum<file>, "error out"=w1980:errorcluster)  [unwired: 1 in]
        n536 = Close File(refnum=w1979, error in=w1980) -> (error out=w1968:errorcluster)  [unwired: 1 out]
      }
      frame "serial" {
        n537 = local read "Termination char\n(0xA = '\\n' = LF)\n(0xD = '\\r' = CR)"() -> (w2043:u8)
        n538 = local read "Enable Termination\nChar (T)"() -> (w2044:bool)
        n539 = Index Array(array=w2051, index=0 ("Index")) -> (element=w2050:string)
        n540 = local read "parity"() -> (w2034:u16)
        n541 = local read "Delay before read (ms)"() -> (w2045:u32)
        n542 = local read "byte count"() -> (w2042:u32)
        n543 = local read "Timeout (ms)"() -> (w2041:u32)
        n544 = local read "VISA resource name"() -> (w2038:refnum<visa-resource-name>)
        n545 = local read "baud rate"() -> (w2037:u32)
        n546 = local read "Serial End Mode for Reads"() -> (w2036:u16)
        n547 = local read "data bits"() -> (w2035:u16)
        n548 = local read "stop bits"() -> (w2040:u16)
        n549 = local read "flow control"() -> (w2039:u16)
        n550 = call "Serial write and read v0.5.vi"("Delay before read (ms)"=w2045, "Termination char\n(0xA = '\\n' = LF)\n(0xD = '\\r' = CR)"=w2043, "Enable Termination\nChar (T)"=w2044, "parity"=w2034, "stop bits"=w2040, "string to write"=w2050, "flow control"=w2039, "byte count"=w2042, "Serial Settings:Serial End Mode for Reads"=w2036, "Timeout (ms)"=w2041, "error in (no error)"=w2056, "VISA resource name"=w2038, "baud rate"=w2037, "data bits"=w2035) -> ("Serial port output"=w2046:string, "error out"=w2055:errorcluster)
        n551 = Build Array (concatenate)(w2046, w2047) -> (w2048:string[])
      }
    }
    n552 = local read "Time Units"() -> (w97:u16)
    n553 = case shown="0" w97 {
      tunnel: ["Time (Seconds)" ("element") "Time (Minutes)" ("element") "Time (Hours)" ("element")] -> w64
      frame 0 {
      }
      frame 1, Default {
      }
      frame 2 {
      }
    }
    n554 = Build Array(w146, w103, w113, w112, w111, w110, w109, w108, w107, w106, w105, w104, w102) -> (w167:dbl[][])
    n555 = Transpose 2D Array(2D array=w167) -> (transposed array=w166:dbl[][])
    n556 = Concatenate Strings(w70, "-I-vs-time.txt" ("Suffix (Imax,Imin,Ion,Ioff)")) -> (w177:string)
    n557 = Build Array(w64, "Is max (A)" ("VAR2 Name"), "Is min (A)" ("VAR2 Name"), "Id max (A)" ("VAR2 Name"), "Id min (A)" ("VAR2 Name"), "Ig max (A)" ("VAR2 Name"), "Ig min (A)" ("VAR2 Name"), "Is on (A)" ("VAR2 Name"), "Is off (A)" ("VAR2 Name"), "Id on (A)" ("VAR2 Name"), "Id off (A)" ("VAR2 Name"), "Ig on (A)" ("VAR2 Name"), "Ig off (A)" ("VAR2 Name")) -> (w172:string[])
    n558 = Array To Spreadsheet String(array=w166, 3:"%e" ("format string")) -> (spreadsheet string=w170:string)  [unwired: 1 in]
    n559 = Array To Spreadsheet String(array=w172, 3:"" ("format string")) -> (spreadsheet string=w171:string)  [unwired: 1 in]
    n560 = String To Path(string=w177) -> (path=w176:path)
    n561 = Build Array(w171, w170) -> (w169:string[])
    n562 = Write to Text File(file (use dialog)=w176, text=w169, error in=w145) -> (refnum out=w178:refnum<file>, error out=w168:errorcluster)  [unwired: 1 in, 1 out]
    n563 = Close File(refnum=w178, error in=w168) -> (error out=w100:errorcluster)  [unwired: 1 out]
    n564 = Concatenate Strings(w70, "-serial-port.txt" ("Suffix (serial port log)")) -> (w148:string)
    n565 = String To Path(string=w148) -> (path=w147:path)
    n566 = Build Array(w64, "Serial port input" ("VAR2 Name"), "Serial port output: ") -> (w138:string[])
    n567 = Array To Spreadsheet String(array=w142, 3:"" ("format string")) -> (spreadsheet string=w135:string)  [unwired: 1 in]
    n568 = Array To Spreadsheet String(array=w138, 3:"" ("format string")) -> (spreadsheet string=w136:string)  [unwired: 1 in]
    n569 = Build Array(w136, w135) -> (w137:string[])
    n570 = Array To Spreadsheet String(array=w141, 3:"" ("format string")) -> (spreadsheet string=w153:string)  [unwired: 1 in]
    n571 = Write to Text File(file (use dialog)=w147, text=w137, error in=w100) -> (refnum out=w149:refnum<file>, error out=w150:errorcluster)  [unwired: 1 in, 1 out]
    n572 = Close File(refnum=w149, error in=w150) -> (error out=w72:errorcluster)  [unwired: 1 out]
    n573 = local write "Serial port data"(w153) -> ()
    n574 = Build Array(w69, w68, w67, w66) -> (w81:dbl[][])
    n575 = Build Array(w64, "Is (A)" ("VAR2 Name"), "Id (A)" ("VAR2 Name"), "Ig (A)" ("VAR2 Name")) -> (w77:string[])
    n576 = Transpose 2D Array(2D array=w81) -> (transposed array=w80:dbl[][])
    n577 = Concatenate Strings(w70, "-sample.txt" ("Suffix (Imax,Imin,Ion,Ioff)")) -> (w87:string)
    n578 = Array To Spreadsheet String(array=w77, 3:"" ("format string")) -> (spreadsheet string=w76:string)  [unwired: 1 in]
    n579 = Array To Spreadsheet String(array=w80, 3:"%e" ("format string")) -> (spreadsheet string=w84:string)  [unwired: 1 in]
    n580 = String To Path(string=w87) -> (path=w86:path)
    n581 = Build Array(w76, w84) -> (w83:string[])
    n582 = Write to Text File(file (use dialog)=w86, text=w83, error in=w72) -> (refnum out=w88:refnum<file>, error out=w82:errorcluster)  [unwired: 1 in, 1 out]
    n583 = Close File(refnum=w88, error in=w82) -> (error out=w71:errorcluster)  [unwired: 1 out]
  }
  "error out" <- w27
  "Timings Indicator" <- w19
  "Probe 4 Indicator" <- w3
  "Is max" <- w13
  "Id max" <- w13
  "Ig max" <- w13
  "Imax vs time" <- w2
  "I vs Vg" <- w2
  "Imin vs time" <- w2
  "I vs Vd" <- w2
  "Serial port data" <- "" ("Serial port data")
  "Is min" <- w12
  "Id min" <- w12
  "Ig min" <- w12
  "Ion vs time" <- w2
  "Ioff vs time" <- w2
  "Is on" <- w11
  "Id on" <- w11
  "Ig on" <- w11
  "Is off" <- w10
  "Id off" <- w10
  "Ig off" <- w10
  "I vs time (Bias Stress)" <- w2
